vi "Main - bkp 2.vi"() -> ()   [LabVIEW 2013]
uses:
  <vilib>/Utility/error.llb/DialogType.ctl
  <vilib>/Utility/miscctls.llb/LVFontTypeDef.ctl
panel:
  out "TctrlConID":refnum<k5>
  out "Error BuvVIctrl":string[](array[string])
  in  "Num of Buvs":u8
  out "BuvCtrlVI_VIRef":refnum<vi>[](array[refnum])
  out "BuvNameArr":string[](array[string])
  out "Buv IP":string[](array[string])
  out "Buv con ID":refnum<k5>
  out "LoadPhase":bool
  in  "Tab Control":T1(tab)
  in  "List of channels":i32(listbox)
  in  "ReadFromFile":bool
  in  "WriteToFile":bool
  out "Дата":string
  out "Время":string
  in  "Comm. current %":dbl=0.5 caption="А" min=0.0 max=72.0 step=0.25
  in  "Common curr. dec":bool
  in  "Common curr. inc":bool
  in  "ConnectAll":bool
  in  "DisconnectAll":bool
  in  "Set Output ON All":bool caption="ВЫХОДЫ ИСТОЧНИКОВ"
  out "текущий ист.":u8
  in  "SetCurrent":dbl min=0.0 max=72.0 step=0.1 format="%#.1g"
  in  "SetVoltage":dbl min=0.0 max=30.0 step=0.1 format="%#.1g"
  in  "SetCurrentB":bool
  in  "SetVoltageB":bool
  in  "SetOutputOffB":bool
  in  "SetOutputOnB":bool
  in  "ConnectChannel":bool
  in  "DisconnectChannel":bool
  out "Напор \nобщий":dbl
  out "Cлив \nобщий":dbl
  out "K3":dbl
  out "К2":dbl
  out "К1":dbl
  out "T upd fl":bool
  in  "NewBuvName":string caption="Имя"
  in  "NewBuvIP":string="172.16.21.xx" caption="IP"
  in  "DeleteBuv":bool caption="Удалить БУВ"
  out "текущий ист. БУВ":u8
  in  "SelectedBuvOutVolt":dbl min=0.0 max=1000.0 step=0.1 format="%.1f"
  in  "SelectedBuvSetVolB":bool
  in  "Buv Table":i32(listbox)=-1
  in  "Quit":bool=TRUE
  in  "AddNewBuv":bool caption="Добавить БУВ"
  out "message event":string=" INSTRUCTIONS:\r\rNormal Use:  When using subVIs that incorporate the error in/error out (or error I/O) structure, place this handler where you want to inform the user of an error, typically at the end of the I/O data path, as the last action of the program.  If the error in error? is ERROR, the handler creates a message describing the error and its source.  If the type of dialog = 1 (default), the message is displayed to the user, who can only acknowedge it.  If the type = 2, the user can acknowledge the message or abort execution; aborting a program with active I/O is not recommended.  If the type = 0, no message is displayed; this is used to process the error programmatically, and the error out cluster elements are wired to individual terminals for that reason.  \r\rOther Use:\n\r\nlocal testing.  To test the error code of a subVI or function that does not have the error I/O structure, you can wire its error code and a source string to the local error code and error source inputs.  If error in error? indicates no error and error code is not equal to 0, the local code and source are substituted for the error in values, and error? is set TRUE (ERROR)."
  in  "SelectedBuvOutStateB":bool
  out "message upd":string=" INSTRUCTIONS:\r\rNormal Use:  When using subVIs that incorporate the error in/error out (or error I/O) structure, place this handler where you want to inform the user of an error, typically at the end of the I/O data path, as the last action of the program.  If the error in error? is ERROR, the handler creates a message describing the error and its source.  If the type of dialog = 1 (default), the message is displayed to the user, who can only acknowedge it.  If the type = 2, the user can acknowledge the message or abort execution; aborting a program with active I/O is not recommended.  If the type = 0, no message is displayed; this is used to process the error programmatically, and the error out cluster elements are wired to individual terminals for that reason.  \r\rOther Use:\n\r\nlocal testing.  To test the error code of a subVI or function that does not have the error I/O structure, you can wire its error code and a source string to the local error code and error source inputs.  If error in error? indicates no error and error code is not equal to 0, the local code and source are substituted for the error in values, and error? is set TRUE (ERROR)."
  in  "WriteToFile Buv":bool
  in  "ReadFromFile Buv":bool
  in  "SetCurrentAll":bool
  in  "SetVoltageAll":bool
  in  "Comm. voltage %":dbl caption="%" min=0.0 max=100.0 step=0.5
  in  "Common volt. dec":bool
  in  "Common volt. inc":bool
  in  "DeleteChannel":bool
  in  "AddChannel":bool
  out "CURRENTSET":dbl[](array[numeric])
  out "NAME":string[](array[string])
  out "ADRESS":string[](array[string])
  out "Measure_VI":refnum<vi>[](array[refnum])
  # "ВСЕ ИСТОЧНИКИ"
  # "ИСТОЧНИК №_"
  # "Линзы жесткой фокусировки ЛУ-20"
  # "Выбрана линза:"
  # "ЛЖФ"
  # "Система охлаждения\n квадрупольных линз"
  # "ЛУ-20"
  # "°С"
  # "°С"
  # "°С"
  # "°С"
  # "°С"
  # "Бак \nтеплообменника"
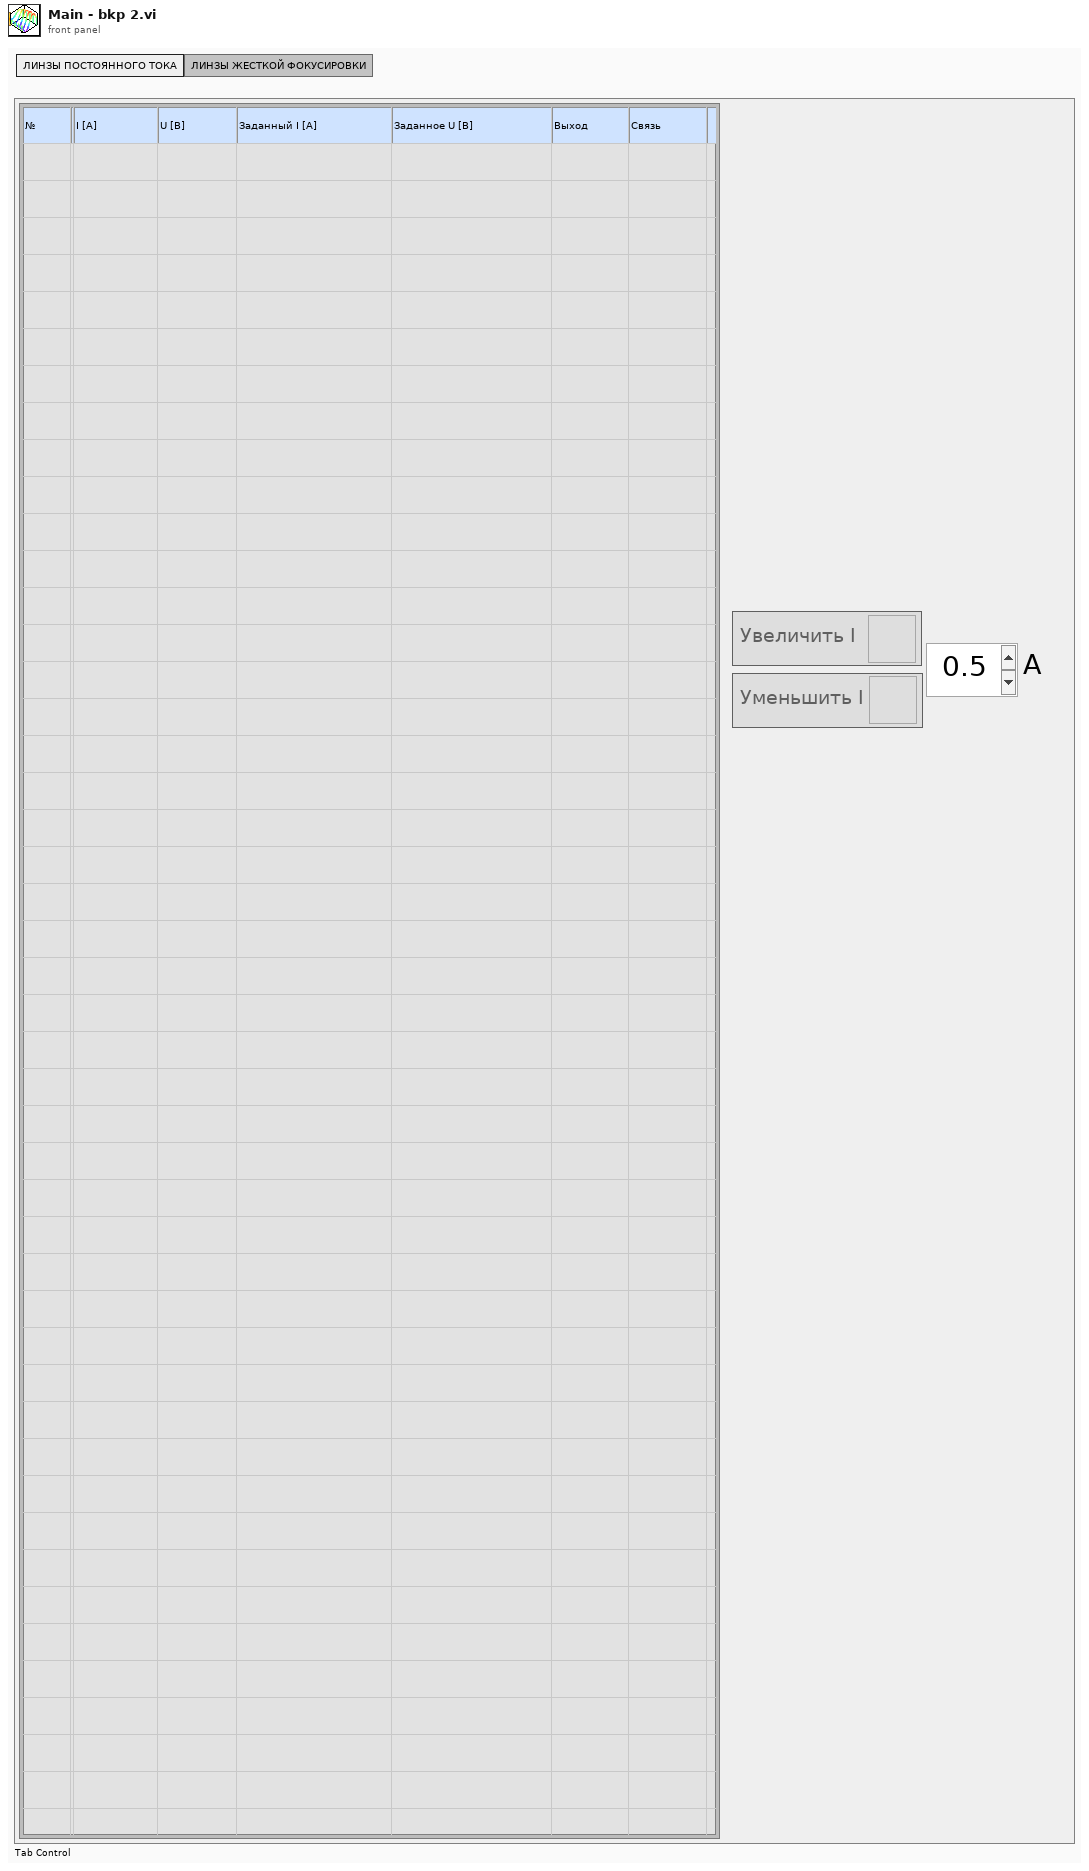
[diagram p1: front panel]
types:
  T1 = enum32{"ЛИНЗЫ ПОСТОЯННОГО ТОКА", "ЛИНЗЫ ЖЕСТКОЙ ФОКУСИРОВКИ"}
  T2 = enum8{"Enabled", "Disabled", "Disabled and Grayed Out"}
  T3 = enum16{"open", "replace", "create", "open or create", "replace or create", "replace or create with confirmation"}
  T4 = typedef "DialogType.ctl" = u16
  T5 = cluster{"T1":dbl, "T2":dbl, "T3":dbl, "T4":dbl, "T5":dbl}
  T6 = cluster{"T 1":bool, "T 2":bool, "T 3":bool, "T 4":bool, "T 5":bool}
  T7 = typedef "LVFontTypeDef.ctl" = cluster{"Font Name":string, "Size":u16, "Bold":bool, "Italic":bool, "Underline":bool, "Strikeout":bool, "Color":u32}
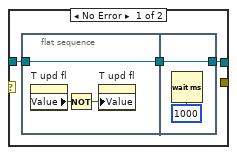
[diagram p2: hidden frame]
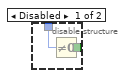
[diagram p4: hidden frame]
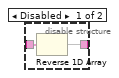
[diagram p6: hidden frame]
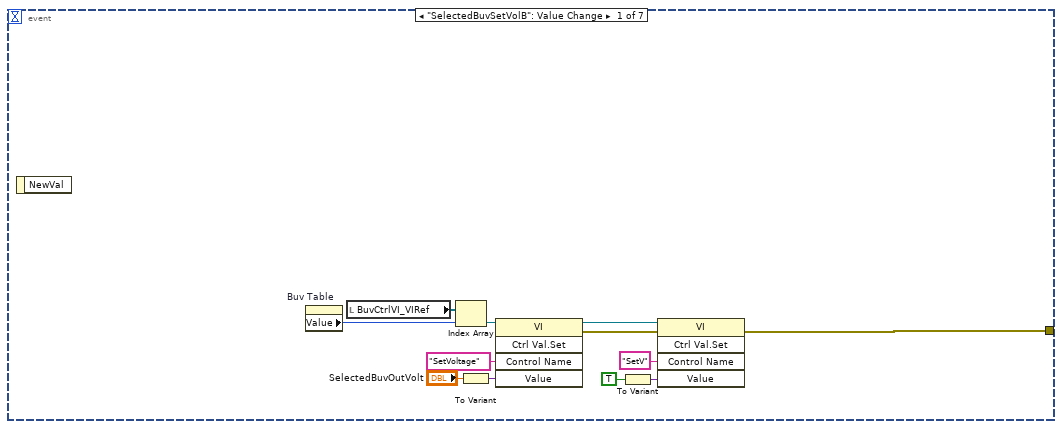
[diagram p7: hidden frame]
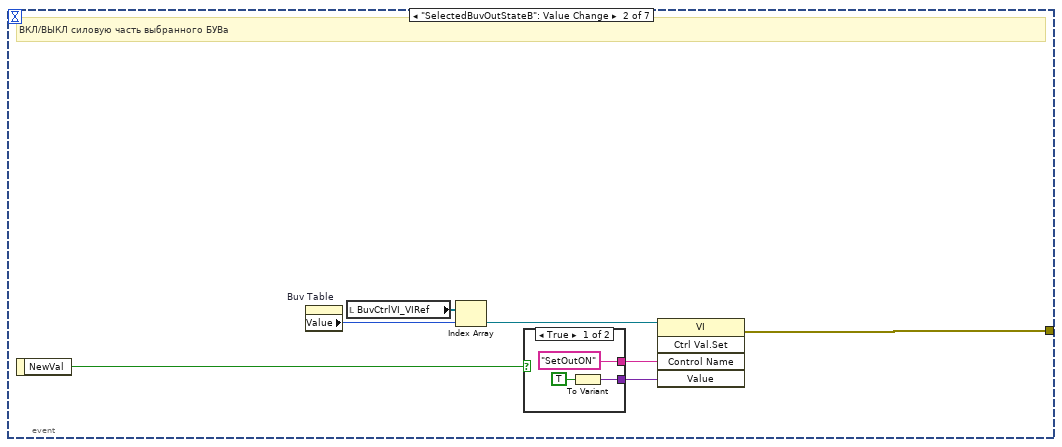
[diagram p8: hidden frame]
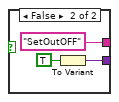
[diagram p9: hidden frame]
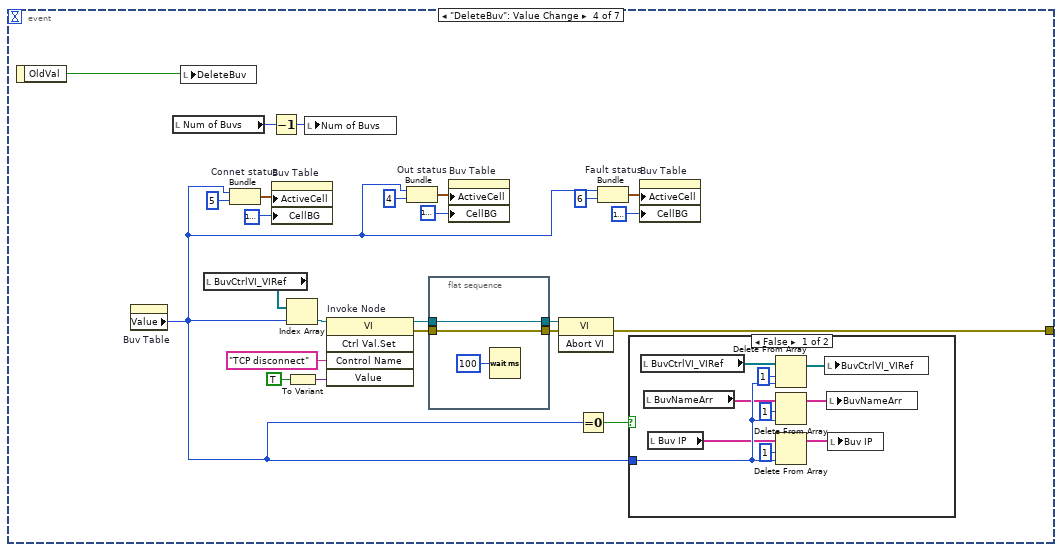
[diagram p10: hidden frame]
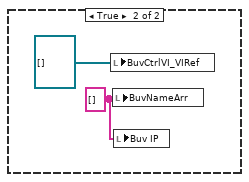
[diagram p11: hidden frame]
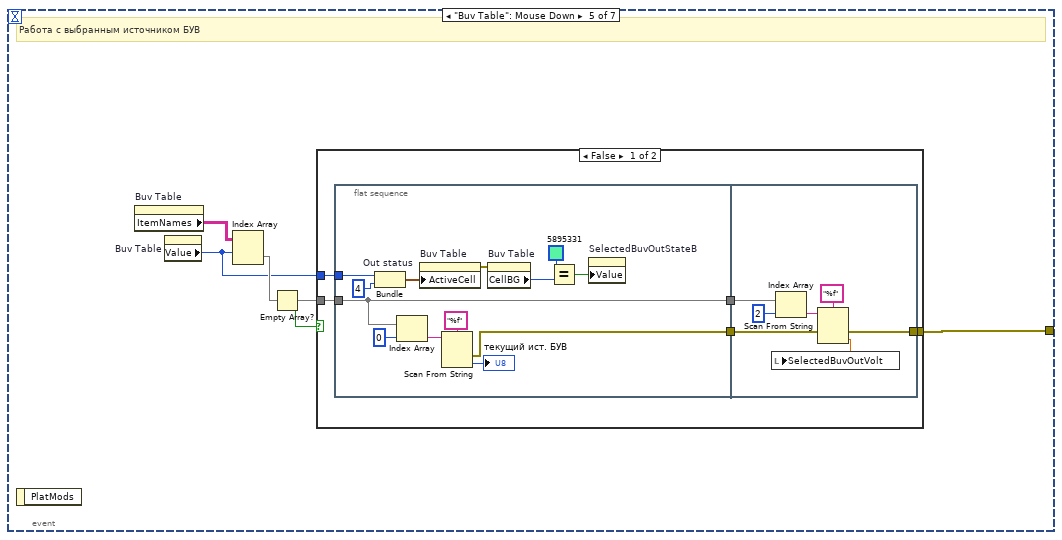
[diagram p12: hidden frame]
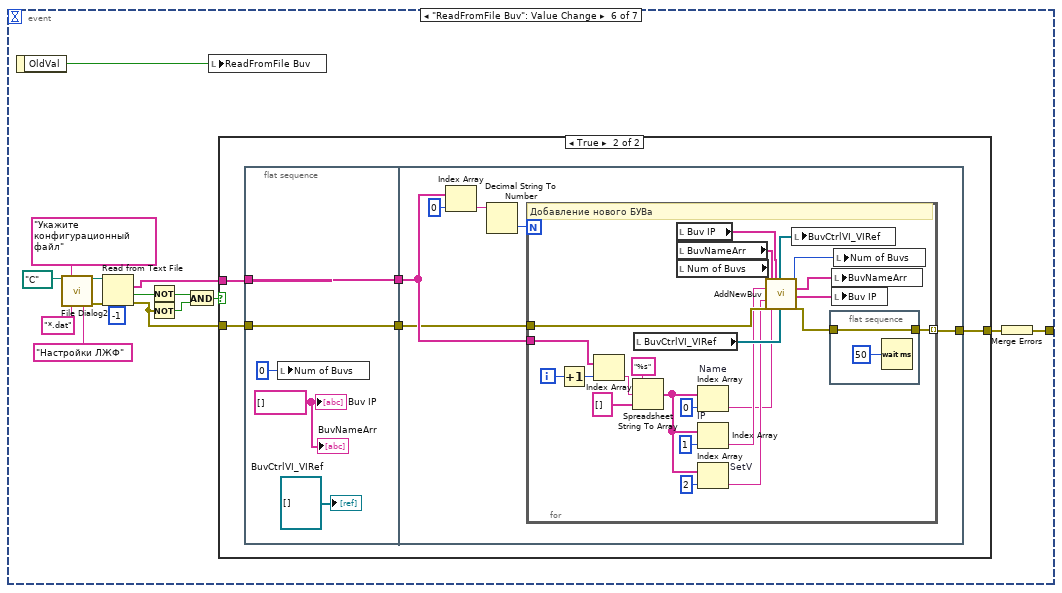
[diagram p14: hidden frame]
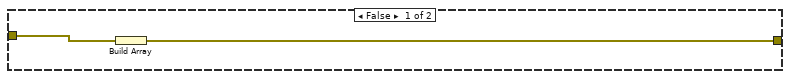
[diagram p15: hidden frame]
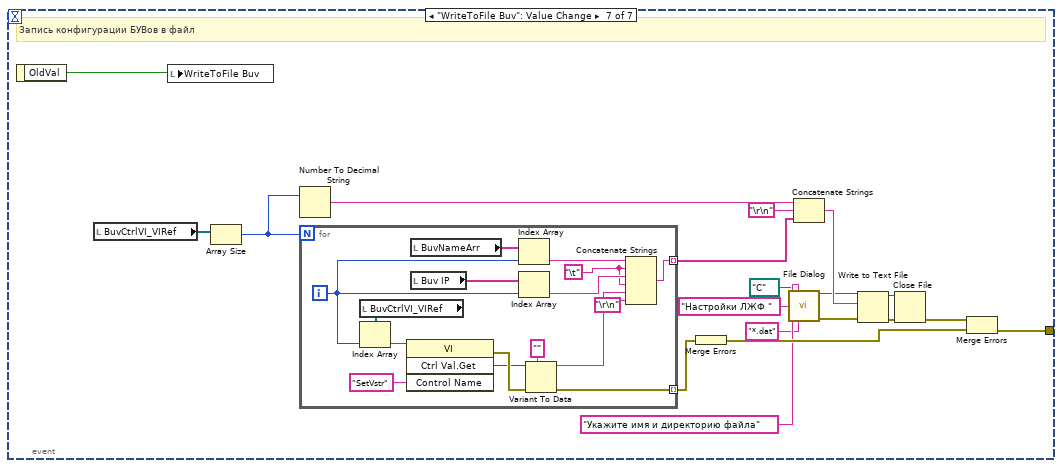
[diagram p16: hidden frame]
diagram:
  w4 = string[] [] ("GlobalInAdress")
  w7 = string[] [] ("GlobalInAdress")
  w24 = u8 0 ("Disabled")
  w8 = FALSE ("SetOutputOnB")
  w26 = FALSE ("OK Button")
  n1 = while {
    stop <- FALSE stop-if-true
    n2 = property on="List of channels" class="MCListbox (strict)"() -> ("ItemNames"=w37:string[][])  [unwired: 2 in, 2 out]
    n3 = Get Date/Time String(want seconds? (F)=TRUE) -> (date string=→"Дата":string, time string=→"Время":string)  [unwired: 2 in]
    n4 = Wait Until Next ms Multiple(millisecond multiple=u16 1000) -> ()  [unwired: 1 out]
    n5 = Empty Array?(array=w37) -> (empty?=w36:bool)
    n6 = case shown="True" w36 {
      tunnel: [T2."Enabled" ("Disabled") T2."Disabled and Grayed Out" ("Disabled")] -> w31
      frame False {
      }
      frame True {
      }
    }
    n7 = property on="Common curr. inc" class="Bool (strict)"("DisabledEnum"=w31) -> ()  [unwired: 2 in, 2 out]
    n8 = property on="Common curr. dec" class="Bool (strict)"("DisabledEnum"=w31) -> ()  [unwired: 2 in, 2 out]
    n9 = property on="Set Output ON All" class="Bool (strict)"("DisabledEnum"=w31) -> ()  [unwired: 2 in, 2 out]
    n10 = property on="Common volt. inc" class="Bool (strict)"("DisabledEnum"=w31) -> ()  [unwired: 2 in, 2 out]
    n11 = property on="DisconnectAll" class="Bool (strict)"("DisabledEnum"=w31) -> ()  [unwired: 2 in, 2 out]
    n12 = property on="SetVoltageB" class="Bool (strict)"("DisabledEnum"=w31) -> ()  [unwired: 2 in, 2 out]
    n13 = property on="ConnectChannel" class="Bool (strict)"("DisabledEnum"=w31) -> ()  [unwired: 2 in, 2 out]
    n14 = property on="SetOutputOnB" class="Bool (strict)"("DisabledEnum"=w31) -> ()  [unwired: 2 in, 2 out]
    n15 = property on="DisconnectChannel" class="Bool (strict)"("DisabledEnum"=w31) -> ()  [unwired: 2 in, 2 out]
    n16 = property on="SetOutputOffB" class="Bool (strict)"("DisabledEnum"=w31) -> ()  [unwired: 2 in, 2 out]
    n17 = property on="ConnectAll" class="Bool (strict)"("DisabledEnum"=w31) -> ()  [unwired: 2 in, 2 out]
    n18 = property on="SetCurrentB" class="Bool (strict)"("DisabledEnum"=w31) -> ()  [unwired: 2 in, 2 out]
  }
  n19 = while {
    stop <- FALSE stop-if-true
    n20 = property on="AddChannel" class="Bool (strict)"() -> ("Disabled"=w48:u8)  [unwired: 2 in, 2 out]
    n21 = Wait Until Next ms Multiple(millisecond multiple=u32 50) -> ()  [unwired: 1 out]
    n22 = local read "Quit"() -> (w46:bool)
    n23 = Not(x=w46) -> (.not. x?=w45:bool)
    n24 = Equal?(x=w48, y=u8 0) -> (x = y?=w44:bool)
    n25 = And(x=w45, y=w44) -> (x .and. y?=w43:bool)
    n26 = case shown="True" w43 {
      frame False {
      }
      frame True {
        w54 = string[] [] ("GlobalInAdress")
        n27 = local read "Measure_VI"() -> (w61:refnum<vi>[])
        n28 = Array Size(array=w61) -> (size(s)=w53:i32)
        n29 = for {
          N: w53 -> [_]
          tunnel: w61 -> [w124]
          shift-right: [w66] -> w52
          shift-left: w54 -> [w63]
          shift-right: [w65] -> w51
          shift-left: w54 -> [w64]
          shift-right: [w115] -> w49
          shift-left: w54 -> [w116]
          shift-right: [w106] -> w50
          shift-left: w54 -> [w111]
          shift-right: [w109] -> w57
          shift-left: w54 -> [w91]
          shift-right: [w104] -> w56
          shift-left: w54 -> [w105]
          i -> [w87]
          w103 = "" ("Control Name")
          n30 = Index Array(array=w124, index=w87) -> (element=w90:refnum<vi>)
          n31 = invoke on="Invoke Node" class="VI" method="Ctrl Val.Get"(reference=w90, "Control Name"="SetVoltageStr") -> (error out=w98:errorcluster, "Get Control Value Variant"=w114:variant)  [unwired: 2 in, 2 out]
          n32 = invoke class="VI" method="Ctrl Val.Get"(reference=w90, "Control Name"="SetCurrentStr") -> (error out=w97:errorcluster, "Get Control Value Variant"=w113:variant)  [unwired: 2 in, 2 out]
          n33 = invoke class="VI" method="Ctrl Val.Get"(reference=w90, "Control Name"="Error") -> (error out=w86:errorcluster, "Get Control Value Variant"=w92:variant)  [unwired: 2 in, 2 out]
          n34 = invoke class="VI" method="Ctrl Val.Get"(reference=w90, "Control Name"="GetCurrent") -> (error out=w100:errorcluster, "Get Control Value Variant"=w121:variant)  [unwired: 2 in, 2 out]
          n35 = invoke class="VI" method="Ctrl Val.Get"(reference=w90, "Control Name"="GetVoltage") -> (error out=w99:errorcluster, "Get Control Value Variant"=w122:variant)  [unwired: 2 in, 2 out]
          n36 = invoke class="VI" method="Ctrl Val.Get"(reference=w90, "Control Name"="Output") -> (error out=w96:errorcluster, "Get Control Value Variant"=w107:variant)  [unwired: 2 in, 2 out]
          n37 = Variant To Data(type=w103, Variant=w114) -> (data=w68:string)  [unwired: 1 in, 1 out]
          n38 = Variant To Data(type=w103, Variant=w113) -> (data=w73:string)  [unwired: 1 in, 1 out]
          n39 = Merge Errors(w86, w100, w99, w98) -> (w95:errorcluster)
          n40 = Variant To Data(type=w103, Variant=w121) -> (data=w118:string)  [unwired: 1 in, 1 out]
          n41 = Variant To Data(type=w103, Variant=w122) -> (data=w119:string)  [unwired: 1 in, 1 out]
          n42 = Variant To Data "Out"(type=w103, Variant=w107) -> (data=w93:string)  [unwired: 1 in, 1 out]
          n43 = Merge Errors(w97, w96) -> (w94:errorcluster)
          n44 = String Length(string=w68) -> (length=w69:i32)
          n45 = String Length(string=w73) -> (length=w76:i32)
          n46 = Variant To Data(type=FALSE, Variant=w92) -> (data=w62:bool)  [unwired: 1 in, 1 out]
          n47 = case shown="False" w62 {
            tunnel: w90 -> [_ w178]
            tunnel: w87 -> [w165 w171]
            tunnel: [w164 w169] -> w83
            frame False {
              n48 = Bundle(w165, "milliseconds to wait"=8) -> (w166:cluster{i32, "milliseconds to wait":i32})  [unwired: 1 in]
              n49 = property on="error" class="MCListbox (strict)"("ActiveCell"=w166, "CellBG"=u32 16777225) -> (error out=w164:errorcluster)  [unwired: 2 in, 1 out]
            }
            frame True {
              n50 = disable-structure shown="Enabled" {
                disable-tunnel: w178 -> [w194 w200]
                disable-tunnel: [w191 _] -> w174
                disable-tunnel: [w189 w200] -> w173
                disable-tunnel: [w187 _] -> w172
                disable-tunnel: w171 -> [w186 w201]
                disable-tunnel: [w185 w201] -> w170
                frame Disabled {
                  w188 = "Connect" ("Control Name")
                  n51 = invoke class="VI" method="Ctrl Val.Set"(reference=w194, "Control Name"=w188, "Value"=FALSE ("OK Button")) -> (reference out=w190:refnum<vi>, error out=w192:errorcluster)  [unwired: 2 in, 3 out]
                  n52 = flat-sequence {
                    tunnel: w192 -> [w199]
                    tunnel: [w199] -> w191
                    tunnel: w190 -> [w197]
                    tunnel: [w197] -> w189
                    tunnel: w188 -> [w196]
                    tunnel: [w196] -> w187
                    tunnel: w186 -> [w195]
                    tunnel: [w195] -> w185
                    frame #0 {
                      n53 = Wait (ms)(milliseconds to wait=u32 2000) -> ()  [unwired: 1 out]
                    }
                  }
                }
                frame Enabled {
                }
              }
              n54 = disable-structure shown="Enabled" {
                disable-tunnel: w174 -> [w182 w184]
                disable-tunnel: w173 -> [w181 _]
                disable-tunnel: w172 -> [w180 _]
                disable-tunnel: [w179 w184] -> w169
                frame Disabled {
                  n55 = invoke class="VI" method="Ctrl Val.Set"(reference=w181, error in=w182, "Control Name"=w180, "Value"=TRUE ("OK Button")) -> (error out=w179:errorcluster)  [unwired: 1 in, 4 out]
                }
                frame Enabled {
                }
              }
              n56 = Bundle(w170, "milliseconds to wait"=8) -> (w175:cluster{i32, "milliseconds to wait":i32})  [unwired: 1 in]
              n57 = property on="error" class="MCListbox (strict)"("ActiveCell"=w175, "CellBG"=u32 16711680) -> ()  [unwired: 2 in, 2 out]
            }
          }
          n58 = case shown="6, Default" w69 {
            tunnel: [4 ("milliseconds to wait") 5 ("milliseconds to wait")] -> w70
            tunnel: [0 ("milliseconds to wait") 0 ("milliseconds to wait")] -> w71
            frame 6, Default {
            }
            frame 7 {
            }
          }
          n59 = case shown="7" w76 {
            tunnel: [4 ("milliseconds to wait") 5 ("milliseconds to wait")] -> w75
            tunnel: [0 ("milliseconds to wait") 0 ("milliseconds to wait")] -> w74
            frame 6, Default {
            }
            frame 7 {
            }
          }
          n60 = Build Array (concatenate)(w63, w118) -> (w66:string[])
          n61 = Build Array (concatenate)(w64, w119) -> (w65:string[])
          n62 = Merge Errors(w95, w94, w83) -> (w89:errorcluster)
          n63 = call <vilib>:"General Error Handler.vi"("type of dialog (OK msg:1)"=u32 0 ("milliseconds to wait"), "error in (no error)"=w89) -> ()  [unwired: 9 in, 5 out]
          n64 = case shown="\"0\"" w93 {
            tunnel: ["+" ("Control Name") "" ("Control Name") "-" ("Control Name")] -> w85
            tunnel: w87 -> [w133 w138 w143]
            frame "1" {
              n65 = Bundle(w133, "milliseconds to wait"=6) -> (w135:cluster{i32, "milliseconds to wait":i32})  [unwired: 1 in]
              n66 = property on="out" class="MCListbox (strict)"("ActiveCell"=w135, "CellBG"=u32 5895331) -> ()  [unwired: 2 in, 2 out]
            }
            frame Default {
              n67 = Bundle(w138, "milliseconds to wait"=6) -> (w140:cluster{i32, "milliseconds to wait":i32})  [unwired: 1 in]
              n68 = property on="out" class="MCListbox (strict)"("ActiveCell"=w140, "CellBG"=u32 16777225) -> ()  [unwired: 2 in, 2 out]
            }
            frame "0" {
              n69 = Bundle(w143, "milliseconds to wait"=6) -> (w145:cluster{i32, "milliseconds to wait":i32})  [unwired: 1 in]
              n70 = property on="out" class="MCListbox (strict)"("ActiveCell"=w145, "CellBG"=u32 13816530) -> ()  [unwired: 2 in, 2 out]
            }
          }
          n71 = String Subset(string=w68, offset (0)=w71, length (rest)=w70) -> (substring=w67:string)
          n72 = String Subset(string=w73, offset (0)=w74, length (rest)=w75) -> (substring=w72:string)
          n73 = case shown="False" w62 {
            tunnel: ["+" ("Control Name") "-" ("Control Name")] -> w110
            tunnel: w87 -> [w149 w156]
            tunnel: w85 -> [w148 _]
            tunnel: [w148 "?" ("Control Name")] -> w84
            frame False {
              n74 = Bundle(w149, "milliseconds to wait"=7) -> (w151:cluster{i32, "milliseconds to wait":i32})  [unwired: 1 in]
              n75 = property on="active" class="MCListbox (strict)"("ActiveCell"=w151, "CellBG"=u32 5895331) -> ()  [unwired: 2 in, 2 out]
            }
            frame True {
              n76 = Bundle(w156, "milliseconds to wait"=7) -> (w162:cluster{i32, "milliseconds to wait":i32})  [unwired: 1 in]
              n77 = property on="active" class="MCListbox (strict)"("ActiveCell"=w162, "CellBG"=u32 14869218) -> (error out=w157:errorcluster)  [unwired: 2 in, 1 out]
              n78 = Bundle(w156, "milliseconds to wait"=6) -> (w155:cluster{i32, "milliseconds to wait":i32})  [unwired: 1 in]
              n79 = property on="out" class="MCListbox (strict)"(error in=w157, "ActiveCell"=w155, "CellBG"=u32 14869218) -> ()  [unwired: 1 in, 2 out]
            }
          }
          n80 = Search and Replace String(input string=w67, search string=",", replace string="." ("replace string (\"\")")) -> (result string=w80:string)  [unwired: 5 in, 3 out]
          n81 = Search and Replace String(input string=w72, search string=",", replace string="." ("replace string (\"\")")) -> (result string=w78:string)  [unwired: 5 in, 3 out]
          n82 = Build Array (concatenate)(w111, w78) -> (w106:string[])
          n83 = Build Array (concatenate)(w116, w80) -> (w115:string[])
          n84 = Build Array (concatenate)(w105, w84) -> (w104:string[])
          n85 = Build Array (concatenate)(w91, w110) -> (w109:string[])
        }
        n86 = local read "ADRESS"() -> (w59:string[])
        n87 = local read "NAME"() -> (w58:string[])
        n88 = Build Array(w58, w59, w52, w51, w50, w49, w56, w57) -> (w60:string[][])
        n89 = Transpose 2D Array(2D array=w60) -> (transposed array=w55:string[][])
        n90 = property on="List of channels" class="MCListbox (strict)"("ItemNames"=w55) -> ()  [unwired: 2 in, 2 out]
      }
    }
  }
  n91 = while {
    stop <- FALSE stop-if-true
    n92 = event shown="[14] \"WriteToFile\": Value Change" {
      selector: _ -> [_ _ _ _ _ _ _ _ _ _ _ _ _ _ _ _ _ _]
      dyn-events: _ -> [_ _ _ _ _ _ _ _ _ _ _ _ _ _ _ _ _ _]
      timeout: _ -> [_ _ _ _ _ _ _ _ _ _ _ _ _ _ _ _ _ _]
      tunnel: [_ _ w272 w288 w304 w345 w386 w401 w427 w443 w459 w476 w497 w520 w538 w589 w667 w690] -> w203
      event "List of channels": Mouse Down {
        # "Работа с выбранным источником"
        n93 = event-data() -> ()  [unwired: 2 out]
        n94 = property on="List of channels" class="MCListbox (strict)"() -> ("ItemNames"=w209:string[][])  [unwired: 2 in, 2 out]
        n95 = property on="List of channels" class="MCListbox (strict)"() -> ("Value"=w208:i32)  [unwired: 2 in, 2 out]
        n96 = Index Array(array=w209, index (row)=w208) -> (element=w207:string[])  [unwired: 1 in]
        n97 = Empty Array?(array=w207) -> (empty?=w206:bool)
        n98 = case shown="False" w206 {
          tunnel: w207 -> [w210 _]
          frame False {
            n99 = flat-sequence {
              tunnel: w210 -> [w216]
              tunnel: [w216] -> w211
              tunnel: w211 -> [w229]
              frame #0 {
                n100 = Index Array(array=w216, index=0) -> (element=w219:string)
                n101 = Index Array(array=w216, index=7) -> (element=w217:string)
                n102 = case shown="\"-\", Default" w217 {
                  tunnel: [T2."Enabled" ("Disabled") T2."Disabled and Grayed Out" ("Disabled")] -> w212
                  tunnel: [w223 w225] -> w213
                  tunnel: [w223 w225] -> w215
                  tunnel: [w223 w225] -> w214
                  frame "-", Default {
                    w223 = T2."Disabled and Grayed Out" ("Disabled")
                  }
                  frame "+" {
                    w225 = T2."Enabled" ("Disabled")
                    # "соединение с ист."
                  }
                }
                n103 = Scan From String(format string="%f", input string=w219) -> (output 1=→"текущий ист.":u8)  [unwired: 3 in, 3 out]
                n104 = property on="DisconnectAll" class="Bool (strict)"("DisabledEnum"=w213) -> ()  [unwired: 2 in, 2 out]
                n105 = property on="DisconnectChannel" class="Bool (strict)"("DisabledEnum"=w213) -> ()  [unwired: 2 in, 2 out]
                n106 = property on="SetOutputOffB" class="Bool (strict)"("DisabledEnum"=w215) -> ()  [unwired: 2 in, 2 out]
                n107 = property on="SetOutputOnB" class="Bool (strict)"("DisabledEnum"=w214) -> ()  [unwired: 2 in, 2 out]
                n108 = property on="ConnectChannel" class="Bool (strict)"("DisabledEnum"=w212) -> ()  [unwired: 2 in, 2 out]
                n109 = property on="ConnectAll" class="Bool (strict)"("DisabledEnum"=w212) -> ()  [unwired: 2 in, 2 out]
              }
              frame #1 {
                n110 = Index Array(array=w229, index=5) -> (element=w234:string)
                n111 = Index Array(array=w229, index=6) -> (element=w237:string)
                n112 = Index Array(array=w229, index=4) -> (element=w231:string)
                n113 = case shown="\"-\", Default" w237 {
                  tunnel: [T2."Enabled" ("Disabled") T2."Disabled and Grayed Out" ("Disabled") w244] -> w238
                  tunnel: [T2."Disabled and Grayed Out" ("Disabled") T2."Enabled" ("Disabled") w244] -> w239
                  frame "-", Default {
                  }
                  frame "+" {
                  }
                  frame "?" {
                    w244 = T2."Disabled and Grayed Out" ("Disabled")
                  }
                }
                n114 = Scan From String(format string="%f", input string=w234) -> (output 1=w227:dbl)  [unwired: 3 in, 3 out]
                n115 = Scan From String(format string="%f", input string=w231) -> (output 1=w228:dbl)  [unwired: 3 in, 3 out]
                n116 = local write "SetVoltage"(w227) -> ()
                n117 = local write "SetCurrent"(w228) -> ()
                n118 = property on="SetOutputOffB" class="Bool (strict)"("DisabledEnum"=w239) -> ()  [unwired: 2 in, 2 out]
                n119 = property on="SetOutputOnB" class="Bool (strict)"("DisabledEnum"=w238) -> ()  [unwired: 2 in, 2 out]
              }
            }
          }
          frame True {
          }
        }
      }
      event Panel Close? {
        n120 = event-data() -> ()  [unwired: 5 out]
        n121 = Two Button Dialog(message="Вы уверены, что хотите закрыть программу?", 1:"Нет" ("F button name (\"Cancel\")"), 2:"Да" ("T button name (\"OK\")")) -> (T button?=w248:bool)
        n122 = case shown="True" w248 {
          frame False {
          }
          frame True {
            n123 = disable-structure shown="Disabled" {
              frame Disabled {
                n124 = local read item#-1() -> (w258)
                n125 = TCP Close Connection(connection ID=w258) -> ()  [unwired: 2 in, 2 out]
              }
              frame Enabled {
              }
            }
            n126 = local read "Measure_VI"() -> (w250:refnum<vi>[])
            n127 = Array Size(array=w250) -> (size(s)=w249:i32)
            n128 = for {
              N: w249 -> [_]
              tunnel: w250 -> [w268]
              tunnel: [w266] -> w257 mode=indexing
              i -> [w269]
              n129 = Index Array(array=w268, index=w269) -> (element=w267:refnum<vi>)
              n130 = invoke class="VI" method="Ctrl Val.Set"(reference=w267, "Control Name"="Connect", "Value"=FALSE) -> (error out=w266:errorcluster)  [unwired: 2 in, 4 out]
            }
            n131 = flat-sequence {
              tunnel: [w260] -> w256
              tunnel: w257 -> [w260]
              frame #0 {
                n132 = Wait (ms)(milliseconds to wait=u32 1000) -> ()  [unwired: 1 out]
              }
            }
            n133 = local read "Measure_VI"() -> (w251:refnum<vi>[])
            n134 = Array Size(array=w251) -> (size(s)=w252:i32)
            n135 = for {
              N: w252 -> [_]
              tunnel: w251 -> [w264]
              tunnel: [w262] -> w253 mode=indexing
              tunnel: w256 -> [w261] mode=indexing
              i -> [w265]
              n136 = Index Array(array=w264, index=w265) -> (element=w263:refnum<vi>)
              n137 = invoke class="VI" method="Abort VI"(reference=w263, error in=w261) -> (error out=w262:errorcluster)  [unwired: 1 in, 2 out]
            }
            n138 = Merge Errors(w253) -> (w254:errorcluster)
            n139 = call <vilib>:"General Error Handler.vi"("type of dialog (OK msg:1)"=u32 0 ("milliseconds to wait"), "error in (no error)"=w254) -> ()  [unwired: 9 in, 5 out]
          }
        }
        n140 = event-data() -> ()  [unwired: 2 in, 1 out]
      }
      event "SetVoltageAll": Value Change {
        n141 = event-data() -> ()  [unwired: 7 out]
        n142 = flat-sequence {
          tunnel: [w276] -> w274
          tunnel: [w285] -> w273
          tunnel: w274 -> [w285]
          frame #0 {
            w275 = u8 2 ("Disabled")
            n143 = property on="Quit" class="Bool (strict)"("Disabled"=w275) -> ()  [unwired: 2 in, 2 out]
            n144 = property on="AddChannel" class="Bool (strict)"("Disabled"=w275) -> ()  [unwired: 2 in, 2 out]
            n145 = property on="DisconnectChannel" class="Bool (strict)"("Disabled"=w275) -> ()  [unwired: 2 in, 2 out]
            n146 = property on="ConnectAll" class="Bool (strict)"("Disabled"=w275) -> ()  [unwired: 2 in, 2 out]
            n147 = property on="ReadFromFile" class="Bool (strict)"("Disabled"=w275) -> ()  [unwired: 2 in, 2 out]
            n148 = property on="ConnectChannel" class="Bool (strict)"("Disabled"=w275) -> ()  [unwired: 2 in, 2 out]
            n149 = property on="DeleteChannel" class="Bool (strict)"("Disabled"=w275) -> ()  [unwired: 2 in, 2 out]
            n150 = property on="SetVoltageB" class="Bool (strict)"("Disabled"=w275) -> ()  [unwired: 2 in, 2 out]
            n151 = property on="Set Output ON All" class="Bool (strict)"("Disabled"=w275) -> ()  [unwired: 2 in, 2 out]
            n152 = property on="SetOutputOffB" class="Bool (strict)"("Disabled"=w275) -> ()  [unwired: 2 in, 2 out]
            n153 = property on="SetVoltageAll" class="Bool (strict)"("Disabled"=w275) -> ()  [unwired: 2 in, 2 out]
            n154 = property on="SetCurrentAll" class="Bool (strict)"("Disabled"=w275) -> ()  [unwired: 2 in, 2 out]
            n155 = property on="DisconnectAll" class="Bool (strict)"("Disabled"=w275) -> ()  [unwired: 2 in, 2 out]
            n156 = property on="WriteToFile" class="Bool (strict)"("Disabled"=w275) -> ()  [unwired: 2 in, 2 out]
            n157 = property on="SetCurrentB" class="Bool (strict)"("Disabled"=w275) -> ()  [unwired: 2 in, 2 out]
            n158 = property on="SetOutputOnB" class="Bool (strict)"("Disabled"=w275) -> ()  [unwired: 2 in, 2 out]
          }
          frame #1 {
            n159 = local read "Measure_VI"() -> (w278:refnum<vi>[])
            n160 = Array Size(array=w278) -> (size(s)=w277:i32)
            n161 = for {
              N: w277 -> [_]
              tunnel: [w279] -> w276 mode=indexing
              i -> [w281]
              n162 = local read "Measure_VI"() -> (w284:refnum<vi>[])
              n163 = Index Array(array=w284, index=w281) -> (element=w280:refnum<vi>)
              n164 = invoke class="VI" method="Ctrl Val.Set"(reference=w280, "Control Name"="NeedToSetVoltage", "Value"=TRUE ("ConnectChannel")) -> (error out=w279:errorcluster)  [unwired: 2 in, 4 out]
            }
          }
          frame #2 {
            w286 = u8 0 ("Disabled")
            n165 = local write "SetVoltageAll"(FALSE ("SetVoltageAll")) -> ()
            n166 = property on="Quit" class="Bool (strict)"("Disabled"=w286) -> ()  [unwired: 2 in, 2 out]
            n167 = property on="AddChannel" class="Bool (strict)"("Disabled"=w286) -> ()  [unwired: 2 in, 2 out]
            n168 = property on="DisconnectChannel" class="Bool (strict)"("Disabled"=w286) -> ()  [unwired: 2 in, 2 out]
            n169 = property on="ReadFromFile" class="Bool (strict)"("Disabled"=w286) -> ()  [unwired: 2 in, 2 out]
            n170 = property on="ConnectChannel" class="Bool (strict)"("Disabled"=w286) -> ()  [unwired: 2 in, 2 out]
            n171 = property on="DeleteChannel" class="Bool (strict)"("Disabled"=w286) -> ()  [unwired: 2 in, 2 out]
            n172 = property on="WriteToFile" class="Bool (strict)"("Disabled"=w286) -> ()  [unwired: 2 in, 2 out]
            n173 = property on="Set Output ON All" class="Bool (strict)"("Disabled"=w286) -> ()  [unwired: 2 in, 2 out]
            n174 = property on="SetCurrentB" class="Bool (strict)"("Disabled"=w286) -> ()  [unwired: 2 in, 2 out]
            n175 = property on="ConnectAll" class="Bool (strict)"("Disabled"=w286) -> ()  [unwired: 2 in, 2 out]
            n176 = property on="SetOutputOnB" class="Bool (strict)"("Disabled"=w286) -> ()  [unwired: 2 in, 2 out]
            n177 = property on="SetVoltageB" class="Bool (strict)"("Disabled"=w286) -> ()  [unwired: 2 in, 2 out]
            n178 = property on="SetOutputOffB" class="Bool (strict)"("Disabled"=w286) -> ()  [unwired: 2 in, 2 out]
            n179 = property on="SetVoltageAll" class="Bool (strict)"("Disabled"=w286) -> ()  [unwired: 2 in, 2 out]
            n180 = property on="SetCurrentAll" class="Bool (strict)"("Disabled"=w286) -> ()  [unwired: 2 in, 2 out]
            n181 = property on="DisconnectAll" class="Bool (strict)"("Disabled"=w286) -> ()  [unwired: 2 in, 2 out]
          }
        }
        n182 = Merge Errors(w273) -> (w272:errorcluster)
      }
      event "SetCurrentAll": Value Change {
        n183 = event-data() -> ()  [unwired: 7 out]
        n184 = flat-sequence {
          tunnel: [w292] -> w290
          tunnel: [w301] -> w289
          tunnel: w290 -> [w301]
          frame #0 {
            w291 = u8 2 ("Disabled")
            n185 = property on="Quit" class="Bool (strict)"("Disabled"=w291) -> ()  [unwired: 2 in, 2 out]
            n186 = property on="AddChannel" class="Bool (strict)"("Disabled"=w291) -> ()  [unwired: 2 in, 2 out]
            n187 = property on="DisconnectChannel" class="Bool (strict)"("Disabled"=w291) -> ()  [unwired: 2 in, 2 out]
            n188 = property on="ConnectAll" class="Bool (strict)"("Disabled"=w291) -> ()  [unwired: 2 in, 2 out]
            n189 = property on="ReadFromFile" class="Bool (strict)"("Disabled"=w291) -> ()  [unwired: 2 in, 2 out]
            n190 = property on="ConnectChannel" class="Bool (strict)"("Disabled"=w291) -> ()  [unwired: 2 in, 2 out]
            n191 = property on="DeleteChannel" class="Bool (strict)"("Disabled"=w291) -> ()  [unwired: 2 in, 2 out]
            n192 = property on="SetOutputOffB" class="Bool (strict)"("Disabled"=w291) -> ()  [unwired: 2 in, 2 out]
            n193 = property on="Set Output ON All" class="Bool (strict)"("Disabled"=w291) -> ()  [unwired: 2 in, 2 out]
            n194 = property on="SetVoltageAll" class="Bool (strict)"("Disabled"=w291) -> ()  [unwired: 2 in, 2 out]
            n195 = property on="SetCurrentAll" class="Bool (strict)"("Disabled"=w291) -> ()  [unwired: 2 in, 2 out]
            n196 = property on="DisconnectAll" class="Bool (strict)"("Disabled"=w291) -> ()  [unwired: 2 in, 2 out]
            n197 = property on="WriteToFile" class="Bool (strict)"("Disabled"=w291) -> ()  [unwired: 2 in, 2 out]
            n198 = property on="SetCurrentB" class="Bool (strict)"("Disabled"=w291) -> ()  [unwired: 2 in, 2 out]
            n199 = property on="SetOutputOnB" class="Bool (strict)"("Disabled"=w291) -> ()  [unwired: 2 in, 2 out]
            n200 = property on="SetVoltageB" class="Bool (strict)"("Disabled"=w291) -> ()  [unwired: 2 in, 2 out]
          }
          frame #1 {
            n201 = local read "Measure_VI"() -> (w294:refnum<vi>[])
            n202 = Array Size(array=w294) -> (size(s)=w293:i32)
            n203 = for {
              N: w293 -> [_]
              tunnel: [w295] -> w292 mode=indexing
              i -> [w297]
              n204 = local read "Measure_VI"() -> (w300:refnum<vi>[])
              n205 = Index Array(array=w300, index=w297) -> (element=w296:refnum<vi>)
              n206 = invoke class="VI" method="Ctrl Val.Set"(reference=w296, "Control Name"="NeedToSetCurrent", "Value"=TRUE ("ConnectChannel")) -> (error out=w295:errorcluster)  [unwired: 2 in, 4 out]
            }
          }
          frame #2 {
            w302 = u8 0 ("Disabled")
            n207 = local write "SetCurrentAll"(FALSE ("SetVoltageAll")) -> ()
            n208 = property on="Quit" class="Bool (strict)"("Disabled"=w302) -> ()  [unwired: 2 in, 2 out]
            n209 = property on="AddChannel" class="Bool (strict)"("Disabled"=w302) -> ()  [unwired: 2 in, 2 out]
            n210 = property on="DisconnectChannel" class="Bool (strict)"("Disabled"=w302) -> ()  [unwired: 2 in, 2 out]
            n211 = property on="ReadFromFile" class="Bool (strict)"("Disabled"=w302) -> ()  [unwired: 2 in, 2 out]
            n212 = property on="ConnectChannel" class="Bool (strict)"("Disabled"=w302) -> ()  [unwired: 2 in, 2 out]
            n213 = property on="DeleteChannel" class="Bool (strict)"("Disabled"=w302) -> ()  [unwired: 2 in, 2 out]
            n214 = property on="WriteToFile" class="Bool (strict)"("Disabled"=w302) -> ()  [unwired: 2 in, 2 out]
            n215 = property on="Set Output ON All" class="Bool (strict)"("Disabled"=w302) -> ()  [unwired: 2 in, 2 out]
            n216 = property on="SetCurrentB" class="Bool (strict)"("Disabled"=w302) -> ()  [unwired: 2 in, 2 out]
            n217 = property on="ConnectAll" class="Bool (strict)"("Disabled"=w302) -> ()  [unwired: 2 in, 2 out]
            n218 = property on="SetOutputOnB" class="Bool (strict)"("Disabled"=w302) -> ()  [unwired: 2 in, 2 out]
            n219 = property on="SetVoltageB" class="Bool (strict)"("Disabled"=w302) -> ()  [unwired: 2 in, 2 out]
            n220 = property on="SetOutputOffB" class="Bool (strict)"("Disabled"=w302) -> ()  [unwired: 2 in, 2 out]
            n221 = property on="SetVoltageAll" class="Bool (strict)"("Disabled"=w302) -> ()  [unwired: 2 in, 2 out]
            n222 = property on="SetCurrentAll" class="Bool (strict)"("Disabled"=w302) -> ()  [unwired: 2 in, 2 out]
            n223 = property on="DisconnectAll" class="Bool (strict)"("Disabled"=w302) -> ()  [unwired: 2 in, 2 out]
          }
        }
        n224 = Merge Errors(w289) -> (w288:errorcluster)
      }
      event "Common curr. inc", "Common curr. dec": Value Change {
        # "Увелич/уменьшение тока на всех ист"
        n225 = event-data() -> ()  [unwired: 2 out]
        n226 = local read "ADRESS"() -> (w307:string[])
        n227 = Array Size(array=w307) -> (size(s)=w308:i32)
        n228 = for {
          N: w308 -> [_]
          tunnel: [w318] -> w306 mode=indexing
          i -> [w332]
          n229 = local read "Measure_VI"() -> (w335:refnum<vi>[])
          n230 = Index Array(array=w335, index=w332) -> (element=w326:refnum<vi>)
          n231 = invoke class="VI" method="Ctrl Val.Get"(reference=w326, "Control Name"="SetCurrentStr") -> (reference out=w320:refnum<vi>, error out=w330:errorcluster, "Get Control Value Variant"=w334:variant)  [unwired: 2 in, 1 out]
          n232 = Variant To Data(error in=w330, type="" ("Control Name"), Variant=w334) -> (data=w329:string, error out=w328:errorcluster)
          n233 = Scan From String(format string="%f", input string=w329, error in=w328) -> (error out=w319:errorcluster, output 1=w317:dbl)  [unwired: 2 in, 2 out]
          n234 = local read "Common curr. inc"() -> (w316:bool)
          n235 = local read "Common curr. dec"() -> (w314:bool)
          n236 = case shown="True" w316 {
            tunnel: "Comm. current %" -> [w340 w344]
            tunnel: w317 -> [w341 w343]
            tunnel: [w341 w342] -> w315
            tunnel: [w340 _] -> w313
            frame False {
            }
            frame True {
              n237 = Add(x=w343, y=w344) -> (x+y=w342:dbl)
            }
          }
          n238 = case shown="True" w314 {
            tunnel: w315 -> [w336 w339]
            tunnel: [w336 w338] -> w312
            tunnel: w313 -> [_ w337]
            frame False {
            }
            frame True {
              n239 = Subtract(x=w339, y=w337) -> (x-y=w338:dbl)
            }
          }
          n240 = invoke class="VI" method="Ctrl Val.Set"(reference=w320, error in=w319, "Control Name"="SetCurrent", "Value"=w312) -> (reference out=w322:refnum<vi>, error out=w321:errorcluster)  [unwired: 1 in, 3 out]
          n241 = invoke class="VI" method="Ctrl Val.Set"(reference=w322, error in=w321, "Control Name"="NeedToSetCurrent", "Value"=TRUE ("ConnectChannel")) -> (error out=w318:errorcluster)  [unwired: 1 in, 4 out]
        }
        n242 = Merge Errors(w306) -> (w305:errorcluster)
        n243 = flat-sequence {
          tunnel: w305 -> [w310]
          tunnel: [w310] -> w304
          frame #0 {
            w309 = FALSE ("ConnectChannel")
            n244 = local write "Common curr. inc"(w309) -> ()
            n245 = local write "Common curr. dec"(w309) -> ()
          }
        }
      }
      event "Common volt. inc", "Common volt. dec": Value Change {
        # "Увелич/уменьшение тока на всех ист"
        n246 = event-data() -> ()  [unwired: 2 out]
        n247 = local read "ADRESS"() -> (w348:string[])
        n248 = Array Size(array=w348) -> (size(s)=w349:i32)
        n249 = for {
          N: w349 -> [_]
          tunnel: [w359] -> w347 mode=indexing
          i -> [w373]
          n250 = local read "Measure_VI"() -> (w376:refnum<vi>[])
          n251 = Index Array(array=w376, index=w373) -> (element=w367:refnum<vi>)
          n252 = invoke class="VI" method="Ctrl Val.Get"(reference=w367, "Control Name"="SetVoltageStr") -> (reference out=w361:refnum<vi>, error out=w371:errorcluster, "Get Control Value Variant"=w375:variant)  [unwired: 2 in, 1 out]
          n253 = Variant To Data(error in=w371, type="" ("Control Name"), Variant=w375) -> (data=w370:string, error out=w369:errorcluster)
          n254 = Scan From String(format string="%f", input string=w370, error in=w369) -> (error out=w360:errorcluster, output 1=w358:dbl)  [unwired: 2 in, 2 out]
          n255 = local read "Common volt. inc"() -> (w357:bool)
          n256 = local read "Common volt. dec"() -> (w355:bool)
          n257 = case shown="True" w357 {
            tunnel: "Comm. voltage %" -> [w381 w385]
            tunnel: w358 -> [w382 w384]
            tunnel: [w382 w383] -> w356
            tunnel: [w381 _] -> w354
            frame False {
            }
            frame True {
              n258 = Add(x=w384, y=w385) -> (x+y=w383:dbl)
            }
          }
          n259 = case shown="False" w355 {
            tunnel: w356 -> [w377 w380]
            tunnel: [w377 w379] -> w353
            tunnel: w354 -> [_ w378]
            frame False {
            }
            frame True {
              n260 = Subtract(x=w380, y=w378) -> (x-y=w379:dbl)
            }
          }
          n261 = invoke class="VI" method="Ctrl Val.Set"(reference=w361, error in=w360, "Control Name"="SetVoltage", "Value"=w353) -> (reference out=w363:refnum<vi>, error out=w362:errorcluster)  [unwired: 1 in, 3 out]
          n262 = invoke class="VI" method="Ctrl Val.Set"(reference=w363, error in=w362, "Control Name"="NeedToSetVoltage", "Value"=TRUE ("ConnectChannel")) -> (error out=w359:errorcluster)  [unwired: 1 in, 4 out]
        }
        n263 = Merge Errors(w347) -> (w346:errorcluster)
        n264 = flat-sequence {
          tunnel: w346 -> [w351]
          tunnel: [w351] -> w345
          frame #0 {
            w350 = FALSE ("ConnectChannel")
            n265 = local write "Common volt. inc"(w350) -> ()
            n266 = local write "Common volt. dec"(w350) -> ()
          }
        }
      }
      event "DisconnectChannel": Value Change {
        n267 = event-data() -> ()  [unwired: 7 out]
        n268 = property on="List of channels" class="MCListbox (strict)"() -> ("Value"=w390:i32)  [unwired: 2 in, 2 out]
        n269 = flat-sequence {
          tunnel: w390 -> [w392]
          tunnel: [w392] -> w389
          tunnel: w389 -> [w394]
          tunnel: [w393] -> w387
          tunnel: [w399] -> w388
          tunnel: w387 -> [w399]
          frame #0 {
            w391 = u8 2 ("Disabled")
            n270 = property on="AddChannel" class="Bool (strict)"("Disabled"=w391) -> ()  [unwired: 2 in, 2 out]
            n271 = property on="Set Output ON All" class="Bool (strict)"("Disabled"=w391) -> ()  [unwired: 2 in, 2 out]
            n272 = property on="ConnectAll" class="Bool (strict)"("Disabled"=w391) -> ()  [unwired: 2 in, 2 out]
            n273 = property on="DisconnectChannel" class="Bool (strict)"("Disabled"=w391) -> ()  [unwired: 2 in, 2 out]
            n274 = property on="ReadFromFile" class="Bool (strict)"("Disabled"=w391) -> ()  [unwired: 2 in, 2 out]
            n275 = property on="Quit" class="Bool (strict)"("Disabled"=w391) -> ()  [unwired: 2 in, 2 out]
            n276 = property on="ConnectChannel" class="Bool (strict)"("Disabled"=w391) -> ()  [unwired: 2 in, 2 out]
            n277 = property on="DeleteChannel" class="Bool (strict)"("Disabled"=w391) -> ()  [unwired: 2 in, 2 out]
            n278 = property on="WriteToFile" class="Bool (strict)"("Disabled"=w391) -> ()  [unwired: 2 in, 2 out]
            n279 = property on="SetCurrentB" class="Bool (strict)"("Disabled"=w391) -> ()  [unwired: 2 in, 2 out]
            n280 = property on="SetOutputOnB" class="Bool (strict)"("Disabled"=w391) -> ()  [unwired: 2 in, 2 out]
            n281 = property on="SetVoltageB" class="Bool (strict)"("Disabled"=w391) -> ()  [unwired: 2 in, 2 out]
            n282 = property on="SetOutputOffB" class="Bool (strict)"("Disabled"=w391) -> ()  [unwired: 2 in, 2 out]
            n283 = property on="SetVoltageAll" class="Bool (strict)"("Disabled"=w391) -> ()  [unwired: 2 in, 2 out]
            n284 = property on="SetCurrentAll" class="Bool (strict)"("Disabled"=w391) -> ()  [unwired: 2 in, 2 out]
            n285 = property on="DisconnectAll" class="Bool (strict)"("Disabled"=w391) -> ()  [unwired: 2 in, 2 out]
          }
          frame #1 {
            w395 = FALSE ("OK Button")
            n286 = local write "DisconnectChannel"(w395) -> ()
            n287 = local read "Measure_VI"() -> (w397:refnum<vi>[])
            n288 = Index Array(array=w397, index=w394) -> (element=w396:refnum<vi>)
            n289 = invoke class="VI" method="Ctrl Val.Set"(reference=w396, "Control Name"="Connect", "Value"=w395) -> (error out=w393:errorcluster)  [unwired: 2 in, 4 out]
          }
          frame #2 {
            w400 = u8 0 ("Disabled")
            n290 = property on="AddChannel" class="Bool (strict)"("Disabled"=w400) -> ()  [unwired: 2 in, 2 out]
            n291 = property on="DisconnectChannel" class="Bool (strict)"("Disabled"=w400) -> ()  [unwired: 2 in, 2 out]
            n292 = property on="ConnectAll" class="Bool (strict)"("Disabled"=w400) -> ()  [unwired: 2 in, 2 out]
            n293 = property on="ReadFromFile" class="Bool (strict)"("Disabled"=w400) -> ()  [unwired: 2 in, 2 out]
            n294 = property on="ConnectChannel" class="Bool (strict)"("Disabled"=w400) -> ()  [unwired: 2 in, 2 out]
            n295 = property on="Quit" class="Bool (strict)"("Disabled"=w400) -> ()  [unwired: 2 in, 2 out]
            n296 = property on="DeleteChannel" class="Bool (strict)"("Disabled"=w400) -> ()  [unwired: 2 in, 2 out]
            n297 = property on="SetOutputOffB" class="Bool (strict)"("Disabled"=w400) -> ()  [unwired: 2 in, 2 out]
            n298 = property on="Set Output ON All" class="Bool (strict)"("Disabled"=w400) -> ()  [unwired: 2 in, 2 out]
            n299 = property on="SetVoltageAll" class="Bool (strict)"("Disabled"=w400) -> ()  [unwired: 2 in, 2 out]
            n300 = property on="SetCurrentAll" class="Bool (strict)"("Disabled"=w400) -> ()  [unwired: 2 in, 2 out]
            n301 = property on="DisconnectAll" class="Bool (strict)"("Disabled"=w400) -> ()  [unwired: 2 in, 2 out]
            n302 = property on="WriteToFile" class="Bool (strict)"("Disabled"=w400) -> ()  [unwired: 2 in, 2 out]
            n303 = property on="SetCurrentB" class="Bool (strict)"("Disabled"=w400) -> ()  [unwired: 2 in, 2 out]
            n304 = property on="SetOutputOnB" class="Bool (strict)"("Disabled"=w400) -> ()  [unwired: 2 in, 2 out]
            n305 = property on="SetVoltageB" class="Bool (strict)"("Disabled"=w400) -> ()  [unwired: 2 in, 2 out]
          }
        }
        n306 = Merge Errors(w388) -> (w386:errorcluster)
      }
      event "ConnectChannel": Value Change {
        n307 = event-data() -> ()  [unwired: 7 out]
        n308 = property on="List of channels" class="MCListbox (strict)"() -> ("Value"=w405:i32)  [unwired: 2 in, 2 out]
        n309 = flat-sequence {
          tunnel: w405 -> [w407]
          tunnel: [w407] -> w404
          tunnel: w404 -> [w412]
          tunnel: [w411] -> w402
          tunnel: [w424] -> w403
          tunnel: w402 -> [w424]
          frame #0 {
            w406 = u8 2 ("Disabled")
            n310 = property on="AddChannel" class="Bool (strict)"("Disabled"=w406) -> ()  [unwired: 2 in, 2 out]
            n311 = property on="Set Output ON All" class="Bool (strict)"("Disabled"=w406) -> ()  [unwired: 2 in, 2 out]
            n312 = property on="ConnectAll" class="Bool (strict)"("Disabled"=w406) -> ()  [unwired: 2 in, 2 out]
            n313 = property on="DisconnectChannel" class="Bool (strict)"("Disabled"=w406) -> ()  [unwired: 2 in, 2 out]
            n314 = property on="ReadFromFile" class="Bool (strict)"("Disabled"=w406) -> ()  [unwired: 2 in, 2 out]
            n315 = property on="Quit" class="Bool (strict)"("Disabled"=w406) -> ()  [unwired: 2 in, 2 out]
            n316 = property on="ConnectChannel" class="Bool (strict)"("Disabled"=w406) -> ()  [unwired: 2 in, 2 out]
            n317 = property on="DeleteChannel" class="Bool (strict)"("Disabled"=w406) -> ()  [unwired: 2 in, 2 out]
            n318 = property on="WriteToFile" class="Bool (strict)"("Disabled"=w406) -> ()  [unwired: 2 in, 2 out]
            n319 = property on="SetCurrentB" class="Bool (strict)"("Disabled"=w406) -> ()  [unwired: 2 in, 2 out]
            n320 = property on="SetOutputOnB" class="Bool (strict)"("Disabled"=w406) -> ()  [unwired: 2 in, 2 out]
            n321 = property on="SetVoltageB" class="Bool (strict)"("Disabled"=w406) -> ()  [unwired: 2 in, 2 out]
            n322 = property on="SetOutputOffB" class="Bool (strict)"("Disabled"=w406) -> ()  [unwired: 2 in, 2 out]
            n323 = property on="SetVoltageAll" class="Bool (strict)"("Disabled"=w406) -> ()  [unwired: 2 in, 2 out]
            n324 = property on="SetCurrentAll" class="Bool (strict)"("Disabled"=w406) -> ()  [unwired: 2 in, 2 out]
            n325 = property on="DisconnectAll" class="Bool (strict)"("Disabled"=w406) -> ()  [unwired: 2 in, 2 out]
          }
          frame #1 {
            n326 = local read "Measure_VI"() -> (w413:refnum<vi>[])
            n327 = Index Array(array=w413, index=w412) -> (element=w410:refnum<vi>)
            n328 = flat-sequence {
              tunnel: w410 -> [w415]
              tunnel: [w414] -> w408
              tunnel: [w418] -> w409
              tunnel: w408 -> [w418]
              tunnel: [w420] -> w411
              tunnel: w409 -> [w421]
              frame #0 {
                n329 = invoke class="VI" method="Ctrl Val.Set"(reference=w415, "Control Name"="Connect", "Value"=FALSE ("OK Button")) -> (reference out=w414:refnum<vi>)  [unwired: 2 in, 4 out]
              }
              frame #1 {
                n330 = Wait (ms)(milliseconds to wait=u32 1000) -> ()  [unwired: 1 out]
              }
              frame #2 {
                n331 = invoke class="VI" method="Ctrl Val.Set"(reference=w421, "Control Name"="Connect", "Value"=TRUE ("OK Button")) -> (error out=w420:errorcluster)  [unwired: 2 in, 4 out]
              }
            }
          }
          frame #2 {
            w425 = u8 0 ("Disabled")
            n332 = local write "ConnectChannel"(FALSE ("ConnectChannel")) -> ()
            n333 = property on="ConnectAll" class="Bool (strict)"("Disabled"=w425) -> ()  [unwired: 2 in, 2 out]
            n334 = property on="Set Output ON All" class="Bool (strict)"("Disabled"=w425) -> ()  [unwired: 2 in, 2 out]
            n335 = property on="AddChannel" class="Bool (strict)"("Disabled"=w425) -> ()  [unwired: 2 in, 2 out]
            n336 = property on="DisconnectChannel" class="Bool (strict)"("Disabled"=w425) -> ()  [unwired: 2 in, 2 out]
            n337 = property on="ReadFromFile" class="Bool (strict)"("Disabled"=w425) -> ()  [unwired: 2 in, 2 out]
            n338 = property on="ConnectChannel" class="Bool (strict)"("Disabled"=w425) -> ()  [unwired: 2 in, 2 out]
            n339 = property on="Quit" class="Bool (strict)"("Disabled"=w425) -> ()  [unwired: 2 in, 2 out]
            n340 = property on="DeleteChannel" class="Bool (strict)"("Disabled"=w425) -> ()  [unwired: 2 in, 2 out]
            n341 = property on="WriteToFile" class="Bool (strict)"("Disabled"=w425) -> ()  [unwired: 2 in, 2 out]
            n342 = property on="SetCurrentB" class="Bool (strict)"("Disabled"=w425) -> ()  [unwired: 2 in, 2 out]
            n343 = property on="SetOutputOnB" class="Bool (strict)"("Disabled"=w425) -> ()  [unwired: 2 in, 2 out]
            n344 = property on="SetVoltageB" class="Bool (strict)"("Disabled"=w425) -> ()  [unwired: 2 in, 2 out]
            n345 = property on="SetOutputOffB" class="Bool (strict)"("Disabled"=w425) -> ()  [unwired: 2 in, 2 out]
            n346 = property on="SetVoltageAll" class="Bool (strict)"("Disabled"=w425) -> ()  [unwired: 2 in, 2 out]
            n347 = property on="SetCurrentAll" class="Bool (strict)"("Disabled"=w425) -> ()  [unwired: 2 in, 2 out]
            n348 = property on="DisconnectAll" class="Bool (strict)"("Disabled"=w425) -> ()  [unwired: 2 in, 2 out]
          }
        }
        n349 = Merge Errors(w403) -> (w401:errorcluster)
      }
      event "ConnectAll": Value Change {
        n350 = event-data() -> ()  [unwired: 7 out]
        n351 = flat-sequence {
          tunnel: [w431] -> w428
          tunnel: [w440] -> w429
          tunnel: w428 -> [w440]
          frame #0 {
            w430 = u8 2 ("Disabled")
            n352 = property on="Quit" class="Bool (strict)"("Disabled"=w430) -> ()  [unwired: 2 in, 2 out]
            n353 = property on="ReadFromFile" class="Bool (strict)"("Disabled"=w430) -> ()  [unwired: 2 in, 2 out]
            n354 = property on="WriteToFile" class="Bool (strict)"("Disabled"=w430) -> ()  [unwired: 2 in, 2 out]
            n355 = property on="ConnectAll" class="Bool (strict)"("Disabled"=w430) -> ()  [unwired: 2 in, 2 out]
            n356 = property on="Set Output ON All" class="Bool (strict)"("Disabled"=w430) -> ()  [unwired: 2 in, 2 out]
            n357 = property on="SetOutputOffB" class="Bool (strict)"("Disabled"=w430) -> ()  [unwired: 2 in, 2 out]
            n358 = property on="AddChannel" class="Bool (strict)"("Disabled"=w430) -> ()  [unwired: 2 in, 2 out]
            n359 = property on="DisconnectChannel" class="Bool (strict)"("Disabled"=w430) -> ()  [unwired: 2 in, 2 out]
            n360 = property on="SetCurrentAll" class="Bool (strict)"("Disabled"=w430) -> ()  [unwired: 2 in, 2 out]
            n361 = property on="SetOutputOnB" class="Bool (strict)"("Disabled"=w430) -> ()  [unwired: 2 in, 2 out]
            n362 = property on="ConnectChannel" class="Bool (strict)"("Disabled"=w430) -> ()  [unwired: 2 in, 2 out]
            n363 = property on="DeleteChannel" class="Bool (strict)"("Disabled"=w430) -> ()  [unwired: 2 in, 2 out]
            n364 = property on="SetCurrentB" class="Bool (strict)"("Disabled"=w430) -> ()  [unwired: 2 in, 2 out]
            n365 = property on="SetVoltageB" class="Bool (strict)"("Disabled"=w430) -> ()  [unwired: 2 in, 2 out]
            n366 = property on="SetVoltageAll" class="Bool (strict)"("Disabled"=w430) -> ()  [unwired: 2 in, 2 out]
            n367 = property on="DisconnectAll" class="Bool (strict)"("Disabled"=w430) -> ()  [unwired: 2 in, 2 out]
          }
          frame #1 {
            n368 = local read "Measure_VI"() -> (w433:refnum<vi>[])
            n369 = Array Size(array=w433) -> (size(s)=w432:i32)
            n370 = for {
              N: w432 -> [_]
              tunnel: [w434] -> w431 mode=indexing
              i -> [w435]
              n371 = local read "Measure_VI"() -> (w438:refnum<vi>[])
              n372 = Index Array(array=w438, index=w435) -> (element=w437:refnum<vi>)
              n373 = invoke class="VI" method="Ctrl Val.Set"(reference=w437, "Control Name"="Connect", "Value"=TRUE ("OK Button")) -> (error out=w434:errorcluster)  [unwired: 2 in, 4 out]
            }
          }
          frame #2 {
            w441 = u8 0 ("Disabled")
            n374 = local write "ConnectAll"(FALSE ("ConnectChannel")) -> ()
            n375 = property on="Quit" class="Bool (strict)"("Disabled"=w441) -> ()  [unwired: 2 in, 2 out]
            n376 = property on="AddChannel" class="Bool (strict)"("Disabled"=w441) -> ()  [unwired: 2 in, 2 out]
            n377 = property on="DisconnectChannel" class="Bool (strict)"("Disabled"=w441) -> ()  [unwired: 2 in, 2 out]
            n378 = property on="ConnectAll" class="Bool (strict)"("Disabled"=w441) -> ()  [unwired: 2 in, 2 out]
            n379 = property on="Set Output ON All" class="Bool (strict)"("Disabled"=w441) -> ()  [unwired: 2 in, 2 out]
            n380 = property on="SetOutputOffB" class="Bool (strict)"("Disabled"=w441) -> ()  [unwired: 2 in, 2 out]
            n381 = property on="SetCurrentAll" class="Bool (strict)"("Disabled"=w441) -> ()  [unwired: 2 in, 2 out]
            n382 = property on="ConnectChannel" class="Bool (strict)"("Disabled"=w441) -> ()  [unwired: 2 in, 2 out]
            n383 = property on="SetVoltageAll" class="Bool (strict)"("Disabled"=w441) -> ()  [unwired: 2 in, 2 out]
            n384 = property on="SetOutputOnB" class="Bool (strict)"("Disabled"=w441) -> ()  [unwired: 2 in, 2 out]
            n385 = property on="DisconnectAll" class="Bool (strict)"("Disabled"=w441) -> ()  [unwired: 2 in, 2 out]
            n386 = property on="ReadFromFile" class="Bool (strict)"("Disabled"=w441) -> ()  [unwired: 2 in, 2 out]
            n387 = property on="WriteToFile" class="Bool (strict)"("Disabled"=w441) -> ()  [unwired: 2 in, 2 out]
            n388 = property on="SetCurrentB" class="Bool (strict)"("Disabled"=w441) -> ()  [unwired: 2 in, 2 out]
            n389 = property on="SetVoltageB" class="Bool (strict)"("Disabled"=w441) -> ()  [unwired: 2 in, 2 out]
            n390 = property on="DeleteChannel" class="Bool (strict)"("Disabled"=w441) -> ()  [unwired: 2 in, 2 out]
          }
        }
        n391 = Merge Errors(w429) -> (w427:errorcluster)
      }
      event "DisconnectAll": Value Change {
        n392 = event-data() -> ()  [unwired: 7 out]
        n393 = flat-sequence {
          tunnel: [w447] -> w445
          tunnel: [w456] -> w444
          tunnel: w445 -> [w456]
          frame #0 {
            w446 = u8 2 ("Disabled")
            n394 = property on="Quit" class="Bool (strict)"("Disabled"=w446) -> ()  [unwired: 2 in, 2 out]
            n395 = property on="ReadFromFile" class="Bool (strict)"("Disabled"=w446) -> ()  [unwired: 2 in, 2 out]
            n396 = property on="ConnectAll" class="Bool (strict)"("Disabled"=w446) -> ()  [unwired: 2 in, 2 out]
            n397 = property on="ConnectChannel" class="Bool (strict)"("Disabled"=w446) -> ()  [unwired: 2 in, 2 out]
            n398 = property on="AddChannel" class="Bool (strict)"("Disabled"=w446) -> ()  [unwired: 2 in, 2 out]
            n399 = property on="DisconnectChannel" class="Bool (strict)"("Disabled"=w446) -> ()  [unwired: 2 in, 2 out]
            n400 = property on="Set Output ON All" class="Bool (strict)"("Disabled"=w446) -> ()  [unwired: 2 in, 2 out]
            n401 = property on="WriteToFile" class="Bool (strict)"("Disabled"=w446) -> ()  [unwired: 2 in, 2 out]
            n402 = property on="SetOutputOffB" class="Bool (strict)"("Disabled"=w446) -> ()  [unwired: 2 in, 2 out]
            n403 = property on="SetCurrentAll" class="Bool (strict)"("Disabled"=w446) -> ()  [unwired: 2 in, 2 out]
            n404 = property on="SetOutputOnB" class="Bool (strict)"("Disabled"=w446) -> ()  [unwired: 2 in, 2 out]
            n405 = property on="DeleteChannel" class="Bool (strict)"("Disabled"=w446) -> ()  [unwired: 2 in, 2 out]
            n406 = property on="SetCurrentB" class="Bool (strict)"("Disabled"=w446) -> ()  [unwired: 2 in, 2 out]
            n407 = property on="SetVoltageB" class="Bool (strict)"("Disabled"=w446) -> ()  [unwired: 2 in, 2 out]
            n408 = property on="SetVoltageAll" class="Bool (strict)"("Disabled"=w446) -> ()  [unwired: 2 in, 2 out]
            n409 = property on="DisconnectAll" class="Bool (strict)"("Disabled"=w446) -> ()  [unwired: 2 in, 2 out]
          }
          frame #1 {
            n410 = local read "Measure_VI"() -> (w449:refnum<vi>[])
            n411 = Array Size(array=w449) -> (size(s)=w448:i32)
            n412 = for {
              N: w448 -> [_]
              tunnel: [w450] -> w447 mode=indexing
              i -> [w451]
              n413 = local read "Measure_VI"() -> (w454:refnum<vi>[])
              n414 = Index Array(array=w454, index=w451) -> (element=w453:refnum<vi>)
              n415 = invoke class="VI" method="Ctrl Val.Set"(reference=w453, "Control Name"="Connect", "Value"=FALSE ("OK Button")) -> (error out=w450:errorcluster)  [unwired: 2 in, 4 out]
            }
          }
          frame #2 {
            w457 = u8 0 ("Disabled")
            n416 = local write "DisconnectAll"(FALSE ("ConnectChannel")) -> ()
            n417 = property on="Quit" class="Bool (strict)"("Disabled"=w457) -> ()  [unwired: 2 in, 2 out]
            n418 = property on="ConnectAll" class="Bool (strict)"("Disabled"=w457) -> ()  [unwired: 2 in, 2 out]
            n419 = property on="ConnectChannel" class="Bool (strict)"("Disabled"=w457) -> ()  [unwired: 2 in, 2 out]
            n420 = property on="AddChannel" class="Bool (strict)"("Disabled"=w457) -> ()  [unwired: 2 in, 2 out]
            n421 = property on="DisconnectChannel" class="Bool (strict)"("Disabled"=w457) -> ()  [unwired: 2 in, 2 out]
            n422 = property on="ReadFromFile" class="Bool (strict)"("Disabled"=w457) -> ()  [unwired: 2 in, 2 out]
            n423 = property on="Set Output ON All" class="Bool (strict)"("Disabled"=w457) -> ()  [unwired: 2 in, 2 out]
            n424 = property on="WriteToFile" class="Bool (strict)"("Disabled"=w457) -> ()  [unwired: 2 in, 2 out]
            n425 = property on="SetOutputOnB" class="Bool (strict)"("Disabled"=w457) -> ()  [unwired: 2 in, 2 out]
            n426 = property on="SetCurrentB" class="Bool (strict)"("Disabled"=w457) -> ()  [unwired: 2 in, 2 out]
            n427 = property on="SetVoltageB" class="Bool (strict)"("Disabled"=w457) -> ()  [unwired: 2 in, 2 out]
            n428 = property on="SetVoltageAll" class="Bool (strict)"("Disabled"=w457) -> ()  [unwired: 2 in, 2 out]
            n429 = property on="DisconnectAll" class="Bool (strict)"("Disabled"=w457) -> ()  [unwired: 2 in, 2 out]
            n430 = property on="DeleteChannel" class="Bool (strict)"("Disabled"=w457) -> ()  [unwired: 2 in, 2 out]
            n431 = property on="SetOutputOffB" class="Bool (strict)"("Disabled"=w457) -> ()  [unwired: 2 in, 2 out]
            n432 = property on="SetCurrentAll" class="Bool (strict)"("Disabled"=w457) -> ()  [unwired: 2 in, 2 out]
          }
        }
        n433 = Merge Errors(w444) -> (w443:errorcluster)
      }
      event "SetVoltageB": Value Change {
        n434 = event-data() -> ()  [unwired: 7 out]
        n435 = local write "SetVoltageB"(FALSE ("ConnectChannel")) -> ()
        n436 = flat-sequence {
          tunnel: [w465] -> w461
          tunnel: [w474] -> w460
          tunnel: w461 -> [w474]
          frame #0 {
            w463 = u8 2 ("Disabled")
            n437 = property on="Quit" class="Bool (strict)"("Disabled"=w463) -> ()  [unwired: 2 in, 2 out]
            n438 = property on="AddChannel" class="Bool (strict)"("Disabled"=w463) -> ()  [unwired: 2 in, 2 out]
            n439 = property on="Set Output ON All" class="Bool (strict)"("Disabled"=w463) -> ()  [unwired: 2 in, 2 out]
            n440 = property on="ConnectAll" class="Bool (strict)"("Disabled"=w463) -> ()  [unwired: 2 in, 2 out]
            n441 = property on="DisconnectChannel" class="Bool (strict)"("Disabled"=w463) -> ()  [unwired: 2 in, 2 out]
            n442 = property on="ReadFromFile" class="Bool (strict)"("Disabled"=w463) -> ()  [unwired: 2 in, 2 out]
            n443 = property on="ConnectChannel" class="Bool (strict)"("Disabled"=w463) -> ()  [unwired: 2 in, 2 out]
            n444 = property on="DeleteChannel" class="Bool (strict)"("Disabled"=w463) -> ()  [unwired: 2 in, 2 out]
            n445 = property on="WriteToFile" class="Bool (strict)"("Disabled"=w463) -> ()  [unwired: 2 in, 2 out]
            n446 = property on="SetCurrentB" class="Bool (strict)"("Disabled"=w463) -> ()  [unwired: 2 in, 2 out]
            n447 = property on="SetOutputOnB" class="Bool (strict)"("Disabled"=w463) -> ()  [unwired: 2 in, 2 out]
            n448 = property on="SetVoltageB" class="Bool (strict)"("Disabled"=w463) -> ()  [unwired: 2 in, 2 out]
            n449 = property on="SetOutputOffB" class="Bool (strict)"("Disabled"=w463) -> ()  [unwired: 2 in, 2 out]
            n450 = property on="SetVoltageAll" class="Bool (strict)"("Disabled"=w463) -> ()  [unwired: 2 in, 2 out]
            n451 = property on="SetCurrentAll" class="Bool (strict)"("Disabled"=w463) -> ()  [unwired: 2 in, 2 out]
            n452 = property on="DisconnectAll" class="Bool (strict)"("Disabled"=w463) -> ()  [unwired: 2 in, 2 out]
          }
          frame #1 {
            n453 = property on="List of channels" class="MCListbox (strict)"() -> ("Value"=w464:i32)  [unwired: 2 in, 2 out]
            n454 = local read "Measure_VI"() -> (w472:refnum<vi>[])
            n455 = local read "SetVoltage"() -> (w470:dbl)
            n456 = Index Array(array=w472, index=w464) -> (element=w471:refnum<vi>)
            n457 = invoke class="VI" method="Ctrl Val.Set"(reference=w471, "Control Name"="SetVoltage", "Value"=w470) -> (reference out=w467:refnum<vi>, error out=w466:errorcluster)  [unwired: 2 in, 3 out]
            n458 = invoke class="VI" method="Ctrl Val.Set"(reference=w467, error in=w466, "Control Name"="NeedToSetVoltage", "Value"=TRUE ("ConnectChannel")) -> (error out=w465:errorcluster)  [unwired: 1 in, 4 out]
          }
          frame #2 {
            w475 = u8 0 ("Disabled")
            n459 = property on="Quit" class="Bool (strict)"("Disabled"=w475) -> ()  [unwired: 2 in, 2 out]
            n460 = property on="ConnectAll" class="Bool (strict)"("Disabled"=w475) -> ()  [unwired: 2 in, 2 out]
            n461 = property on="Set Output ON All" class="Bool (strict)"("Disabled"=w475) -> ()  [unwired: 2 in, 2 out]
            n462 = property on="AddChannel" class="Bool (strict)"("Disabled"=w475) -> ()  [unwired: 2 in, 2 out]
            n463 = property on="DisconnectChannel" class="Bool (strict)"("Disabled"=w475) -> ()  [unwired: 2 in, 2 out]
            n464 = property on="ReadFromFile" class="Bool (strict)"("Disabled"=w475) -> ()  [unwired: 2 in, 2 out]
            n465 = property on="ConnectChannel" class="Bool (strict)"("Disabled"=w475) -> ()  [unwired: 2 in, 2 out]
            n466 = property on="DeleteChannel" class="Bool (strict)"("Disabled"=w475) -> ()  [unwired: 2 in, 2 out]
            n467 = property on="SetVoltageAll" class="Bool (strict)"("Disabled"=w475) -> ()  [unwired: 2 in, 2 out]
            n468 = property on="SetCurrentAll" class="Bool (strict)"("Disabled"=w475) -> ()  [unwired: 2 in, 2 out]
            n469 = property on="DisconnectAll" class="Bool (strict)"("Disabled"=w475) -> ()  [unwired: 2 in, 2 out]
            n470 = property on="WriteToFile" class="Bool (strict)"("Disabled"=w475) -> ()  [unwired: 2 in, 2 out]
            n471 = property on="SetCurrentB" class="Bool (strict)"("Disabled"=w475) -> ()  [unwired: 2 in, 2 out]
            n472 = property on="SetOutputOnB" class="Bool (strict)"("Disabled"=w475) -> ()  [unwired: 2 in, 2 out]
            n473 = property on="SetVoltageB" class="Bool (strict)"("Disabled"=w475) -> ()  [unwired: 2 in, 2 out]
            n474 = property on="SetOutputOffB" class="Bool (strict)"("Disabled"=w475) -> ()  [unwired: 2 in, 2 out]
          }
        }
        n475 = Merge Errors(w460) -> (w459:errorcluster)
      }
      event "SetOutputOnB": Value Change {
        n476 = event-data() -> ()  [unwired: 2 out]
        n477 = property on="List of channels" class="MCListbox (strict)"() -> ("Value"=w479:i32)  [unwired: 2 in, 2 out]
        n478 = flat-sequence {
          tunnel: w479 -> [w481]
          tunnel: [w481] -> w478
          tunnel: w478 -> [w488]
          tunnel: [w483] -> w477
          tunnel: [w493] -> w476
          tunnel: w477 -> [w493]
          frame #0 {
            w480 = u8 2 ("Disabled")
            n479 = property on="ConnectAll" class="Bool (strict)"("Disabled"=w480) -> ()  [unwired: 2 in, 2 out]
            n480 = property on="Set Output ON All" class="Bool (strict)"("Disabled"=w480) -> ()  [unwired: 2 in, 2 out]
            n481 = property on="AddChannel" class="Bool (strict)"("Disabled"=w480) -> ()  [unwired: 2 in, 2 out]
            n482 = property on="DisconnectChannel" class="Bool (strict)"("Disabled"=w480) -> ()  [unwired: 2 in, 2 out]
            n483 = property on="ReadFromFile" class="Bool (strict)"("Disabled"=w480) -> ()  [unwired: 2 in, 2 out]
            n484 = property on="Quit" class="Bool (strict)"("Disabled"=w480) -> ()  [unwired: 2 in, 2 out]
            n485 = property on="ConnectChannel" class="Bool (strict)"("Disabled"=w480) -> ()  [unwired: 2 in, 2 out]
            n486 = property on="DeleteChannel" class="Bool (strict)"("Disabled"=w480) -> ()  [unwired: 2 in, 2 out]
            n487 = property on="WriteToFile" class="Bool (strict)"("Disabled"=w480) -> ()  [unwired: 2 in, 2 out]
            n488 = property on="SetCurrentB" class="Bool (strict)"("Disabled"=w480) -> ()  [unwired: 2 in, 2 out]
            n489 = property on="SetOutputOnB" class="Bool (strict)"("Disabled"=w480) -> ()  [unwired: 2 in, 2 out]
            n490 = property on="SetVoltageB" class="Bool (strict)"("Disabled"=w480) -> ()  [unwired: 2 in, 2 out]
            n491 = property on="SetOutputOffB" class="Bool (strict)"("Disabled"=w480) -> ()  [unwired: 2 in, 2 out]
            n492 = property on="SetVoltageAll" class="Bool (strict)"("Disabled"=w480) -> ()  [unwired: 2 in, 2 out]
            n493 = property on="SetCurrentAll" class="Bool (strict)"("Disabled"=w480) -> ()  [unwired: 2 in, 2 out]
            n494 = property on="DisconnectAll" class="Bool (strict)"("Disabled"=w480) -> ()  [unwired: 2 in, 2 out]
          }
          frame #1 {
            n495 = local write "SetOutputOnB"(FALSE ("ConnectChannel")) -> ()
            n496 = local read "Measure_VI"() -> (w491:refnum<vi>[])
            n497 = Index Array(array=w491, index=w488) -> (element=w490:refnum<vi>)
            n498 = invoke class="VI" method="Ctrl Val.Set"(reference=w490, "Control Name"="SetOutput", "Value"=TRUE ("ConnectChannel")) -> (reference out=w485:refnum<vi>, error out=w484:errorcluster)  [unwired: 2 in, 3 out]
            n499 = invoke class="VI" method="Ctrl Val.Set"(reference=w485, error in=w484, "Control Name"="NeedToSetOutput", "Value"=TRUE ("ConnectChannel")) -> (error out=w483:errorcluster)  [unwired: 1 in, 4 out]
          }
          frame #2 {
            w494 = u8 0 ("Disabled")
            n500 = property on="ConnectAll" class="Bool (strict)"("Disabled"=w494) -> ()  [unwired: 2 in, 2 out]
            n501 = property on="Set Output ON All" class="Bool (strict)"("Disabled"=w494) -> ()  [unwired: 2 in, 2 out]
            n502 = property on="AddChannel" class="Bool (strict)"("Disabled"=w494) -> ()  [unwired: 2 in, 2 out]
            n503 = property on="DisconnectChannel" class="Bool (strict)"("Disabled"=w494) -> ()  [unwired: 2 in, 2 out]
            n504 = property on="ReadFromFile" class="Bool (strict)"("Disabled"=w494) -> ()  [unwired: 2 in, 2 out]
            n505 = property on="ConnectChannel" class="Bool (strict)"("Disabled"=w494) -> ()  [unwired: 2 in, 2 out]
            n506 = property on="Quit" class="Bool (strict)"("Disabled"=w494) -> ()  [unwired: 2 in, 2 out]
            n507 = property on="DeleteChannel" class="Bool (strict)"("Disabled"=w494) -> ()  [unwired: 2 in, 2 out]
            n508 = property on="SetOutputOffB" class="Bool (strict)"("Disabled"=w494) -> ()  [unwired: 2 in, 2 out]
            n509 = property on="SetVoltageAll" class="Bool (strict)"("Disabled"=w494) -> ()  [unwired: 2 in, 2 out]
            n510 = property on="SetCurrentAll" class="Bool (strict)"("Disabled"=w494) -> ()  [unwired: 2 in, 2 out]
            n511 = property on="DisconnectAll" class="Bool (strict)"("Disabled"=w494) -> ()  [unwired: 2 in, 2 out]
            n512 = property on="WriteToFile" class="Bool (strict)"("Disabled"=w494) -> ()  [unwired: 2 in, 2 out]
            n513 = property on="SetCurrentB" class="Bool (strict)"("Disabled"=w494) -> ()  [unwired: 2 in, 2 out]
            n514 = property on="SetOutputOnB" class="Bool (strict)"("Disabled"=w494) -> ()  [unwired: 2 in, 2 out]
            n515 = property on="SetVoltageB" class="Bool (strict)"("Disabled"=w494) -> ()  [unwired: 2 in, 2 out]
          }
        }
      }
      event "Set Output ON All": Value Change {
        n516 = event-data() -> ("NewVal"=w495:bool)  [unwired: 1 out]
        n517 = flat-sequence {
          tunnel: [w500] -> w496
          tunnel: w495 -> [w500]
          tunnel: [w505] -> w498
          tunnel: w496 -> [w502]
          tunnel: [w516] -> w499
          tunnel: w498 -> [w516]
          frame #0 {
            w501 = u8 2 ("Disabled")
            n518 = property on="Quit" class="Bool (strict)"("Disabled"=w501) -> ()  [unwired: 2 in, 2 out]
            n519 = property on="AddChannel" class="Bool (strict)"("Disabled"=w501) -> ()  [unwired: 2 in, 2 out]
            n520 = property on="DisconnectChannel" class="Bool (strict)"("Disabled"=w501) -> ()  [unwired: 2 in, 2 out]
            n521 = property on="ConnectAll" class="Bool (strict)"("Disabled"=w501) -> ()  [unwired: 2 in, 2 out]
            n522 = property on="ReadFromFile" class="Bool (strict)"("Disabled"=w501) -> ()  [unwired: 2 in, 2 out]
            n523 = property on="ConnectChannel" class="Bool (strict)"("Disabled"=w501) -> ()  [unwired: 2 in, 2 out]
            n524 = property on="DeleteChannel" class="Bool (strict)"("Disabled"=w501) -> ()  [unwired: 2 in, 2 out]
            n525 = property on="WriteToFile" class="Bool (strict)"("Disabled"=w501) -> ()  [unwired: 2 in, 2 out]
            n526 = property on="SetCurrentB" class="Bool (strict)"("Disabled"=w501) -> ()  [unwired: 2 in, 2 out]
            n527 = property on="SetOutputOnB" class="Bool (strict)"("Disabled"=w501) -> ()  [unwired: 2 in, 2 out]
            n528 = property on="SetVoltageB" class="Bool (strict)"("Disabled"=w501) -> ()  [unwired: 2 in, 2 out]
            n529 = property on="SetOutputOffB" class="Bool (strict)"("Disabled"=w501) -> ()  [unwired: 2 in, 2 out]
            n530 = property on="SetVoltageAll" class="Bool (strict)"("Disabled"=w501) -> ()  [unwired: 2 in, 2 out]
            n531 = property on="SetCurrentAll" class="Bool (strict)"("Disabled"=w501) -> ()  [unwired: 2 in, 2 out]
            n532 = property on="DisconnectAll" class="Bool (strict)"("Disabled"=w501) -> ()  [unwired: 2 in, 2 out]
          }
          frame #1 {
            n533 = local read "Measure_VI"() -> (w504:refnum<vi>[])
            n534 = Array Size(array=w504) -> (size(s)=w503:i32)
            n535 = for {
              N: w503 -> [_]
              tunnel: [w507] -> w505 mode=indexing
              tunnel: w502 -> [w506]
              i -> [w509]
              n536 = local read "Measure_VI"() -> (w514:refnum<vi>[])
              n537 = Index Array(array=w514, index=w509) -> (element=w513:refnum<vi>)
              n538 = invoke class="VI" method="Ctrl Val.Set"(reference=w513, "Control Name"="SetOutput", "Value"=w506) -> (reference out=w510:refnum<vi>, error out=w508:errorcluster)  [unwired: 2 in, 3 out]
              n539 = invoke class="VI" method="Ctrl Val.Set"(reference=w510, error in=w508, "Control Name"="NeedToSetOutput", "Value"=TRUE ("ConnectChannel")) -> (error out=w507:errorcluster)  [unwired: 1 in, 4 out]
            }
          }
          frame #2 {
            w517 = u8 0 ("Disabled")
            n540 = disable-structure shown="Disabled" {
              frame Disabled {
                n541 = local write "Set Output ON All"(FALSE ("ConnectChannel")) -> ()
              }
              frame Enabled {
              }
            }
            n542 = property on="Quit" class="Bool (strict)"("Disabled"=w517) -> ()  [unwired: 2 in, 2 out]
            n543 = property on="ConnectAll" class="Bool (strict)"("Disabled"=w517) -> ()  [unwired: 2 in, 2 out]
            n544 = property on="Set Output ON All" class="Bool (strict)"("Disabled"=w517) -> ()  [unwired: 2 in, 2 out]
            n545 = property on="AddChannel" class="Bool (strict)"("Disabled"=w517) -> ()  [unwired: 2 in, 2 out]
            n546 = property on="DisconnectChannel" class="Bool (strict)"("Disabled"=w517) -> ()  [unwired: 2 in, 2 out]
            n547 = property on="ReadFromFile" class="Bool (strict)"("Disabled"=w517) -> ()  [unwired: 2 in, 2 out]
            n548 = property on="ConnectChannel" class="Bool (strict)"("Disabled"=w517) -> ()  [unwired: 2 in, 2 out]
            n549 = property on="DeleteChannel" class="Bool (strict)"("Disabled"=w517) -> ()  [unwired: 2 in, 2 out]
            n550 = property on="SetVoltageB" class="Bool (strict)"("Disabled"=w517) -> ()  [unwired: 2 in, 2 out]
            n551 = property on="SetOutputOffB" class="Bool (strict)"("Disabled"=w517) -> ()  [unwired: 2 in, 2 out]
            n552 = property on="SetVoltageAll" class="Bool (strict)"("Disabled"=w517) -> ()  [unwired: 2 in, 2 out]
            n553 = property on="SetCurrentAll" class="Bool (strict)"("Disabled"=w517) -> ()  [unwired: 2 in, 2 out]
            n554 = property on="DisconnectAll" class="Bool (strict)"("Disabled"=w517) -> ()  [unwired: 2 in, 2 out]
            n555 = property on="WriteToFile" class="Bool (strict)"("Disabled"=w517) -> ()  [unwired: 2 in, 2 out]
            n556 = property on="SetCurrentB" class="Bool (strict)"("Disabled"=w517) -> ()  [unwired: 2 in, 2 out]
            n557 = property on="SetOutputOnB" class="Bool (strict)"("Disabled"=w517) -> ()  [unwired: 2 in, 2 out]
          }
        }
        n558 = Merge Errors(w499) -> (w497:errorcluster)
      }
      event "SetOutputOffB": Value Change {
        n559 = event-data() -> ()  [unwired: 7 out]
        n560 = local write "SetOutputOffB"(FALSE ("ConnectChannel")) -> ()
        n561 = property on="List of channels" class="MCListbox (strict)"() -> ("Value"=w523:i32)  [unwired: 2 in, 2 out]
        n562 = flat-sequence {
          tunnel: w523 -> [w525]
          tunnel: [w525] -> w522
          tunnel: w522 -> [w532]
          tunnel: [w526] -> w519
          tunnel: [w536] -> w520
          tunnel: w519 -> [w536]
          frame #0 {
            w524 = u8 2 ("Disabled")
            n563 = property on="ConnectAll" class="Bool (strict)"("Disabled"=w524) -> ()  [unwired: 2 in, 2 out]
            n564 = property on="Set Output ON All" class="Bool (strict)"("Disabled"=w524) -> ()  [unwired: 2 in, 2 out]
            n565 = property on="AddChannel" class="Bool (strict)"("Disabled"=w524) -> ()  [unwired: 2 in, 2 out]
            n566 = property on="DisconnectChannel" class="Bool (strict)"("Disabled"=w524) -> ()  [unwired: 2 in, 2 out]
            n567 = property on="ReadFromFile" class="Bool (strict)"("Disabled"=w524) -> ()  [unwired: 2 in, 2 out]
            n568 = property on="Quit" class="Bool (strict)"("Disabled"=w524) -> ()  [unwired: 2 in, 2 out]
            n569 = property on="ConnectChannel" class="Bool (strict)"("Disabled"=w524) -> ()  [unwired: 2 in, 2 out]
            n570 = property on="DeleteChannel" class="Bool (strict)"("Disabled"=w524) -> ()  [unwired: 2 in, 2 out]
            n571 = property on="WriteToFile" class="Bool (strict)"("Disabled"=w524) -> ()  [unwired: 2 in, 2 out]
            n572 = property on="SetCurrentB" class="Bool (strict)"("Disabled"=w524) -> ()  [unwired: 2 in, 2 out]
            n573 = property on="SetOutputOnB" class="Bool (strict)"("Disabled"=w524) -> ()  [unwired: 2 in, 2 out]
            n574 = property on="SetVoltageB" class="Bool (strict)"("Disabled"=w524) -> ()  [unwired: 2 in, 2 out]
            n575 = property on="SetOutputOffB" class="Bool (strict)"("Disabled"=w524) -> ()  [unwired: 2 in, 2 out]
            n576 = property on="SetVoltageAll" class="Bool (strict)"("Disabled"=w524) -> ()  [unwired: 2 in, 2 out]
            n577 = property on="SetCurrentAll" class="Bool (strict)"("Disabled"=w524) -> ()  [unwired: 2 in, 2 out]
            n578 = property on="DisconnectAll" class="Bool (strict)"("Disabled"=w524) -> ()  [unwired: 2 in, 2 out]
          }
          frame #1 {
            n579 = local read "Measure_VI"() -> (w534:refnum<vi>[])
            n580 = Index Array(array=w534, index=w532) -> (element=w533:refnum<vi>)
            n581 = invoke class="VI" method="Ctrl Val.Set"(reference=w533, "Control Name"="SetOutput", "Value"=FALSE ("ConnectChannel")) -> (reference out=w529:refnum<vi>, error out=w527:errorcluster)  [unwired: 2 in, 3 out]
            n582 = invoke class="VI" method="Ctrl Val.Set"(reference=w529, error in=w527, "Control Name"="NeedToSetOutput", "Value"=TRUE ("ConnectChannel")) -> (error out=w526:errorcluster)  [unwired: 1 in, 4 out]
          }
          frame #2 {
            w537 = u8 0 ("Disabled")
            n583 = property on="ConnectAll" class="Bool (strict)"("Disabled"=w537) -> ()  [unwired: 2 in, 2 out]
            n584 = property on="Set Output ON All" class="Bool (strict)"("Disabled"=w537) -> ()  [unwired: 2 in, 2 out]
            n585 = property on="AddChannel" class="Bool (strict)"("Disabled"=w537) -> ()  [unwired: 2 in, 2 out]
            n586 = property on="DisconnectChannel" class="Bool (strict)"("Disabled"=w537) -> ()  [unwired: 2 in, 2 out]
            n587 = property on="ReadFromFile" class="Bool (strict)"("Disabled"=w537) -> ()  [unwired: 2 in, 2 out]
            n588 = property on="ConnectChannel" class="Bool (strict)"("Disabled"=w537) -> ()  [unwired: 2 in, 2 out]
            n589 = property on="Quit" class="Bool (strict)"("Disabled"=w537) -> ()  [unwired: 2 in, 2 out]
            n590 = property on="DeleteChannel" class="Bool (strict)"("Disabled"=w537) -> ()  [unwired: 2 in, 2 out]
            n591 = property on="SetOutputOffB" class="Bool (strict)"("Disabled"=w537) -> ()  [unwired: 2 in, 2 out]
            n592 = property on="SetVoltageAll" class="Bool (strict)"("Disabled"=w537) -> ()  [unwired: 2 in, 2 out]
            n593 = property on="SetCurrentAll" class="Bool (strict)"("Disabled"=w537) -> ()  [unwired: 2 in, 2 out]
            n594 = property on="DisconnectAll" class="Bool (strict)"("Disabled"=w537) -> ()  [unwired: 2 in, 2 out]
            n595 = property on="WriteToFile" class="Bool (strict)"("Disabled"=w537) -> ()  [unwired: 2 in, 2 out]
            n596 = property on="SetCurrentB" class="Bool (strict)"("Disabled"=w537) -> ()  [unwired: 2 in, 2 out]
            n597 = property on="SetOutputOnB" class="Bool (strict)"("Disabled"=w537) -> ()  [unwired: 2 in, 2 out]
            n598 = property on="SetVoltageB" class="Bool (strict)"("Disabled"=w537) -> ()  [unwired: 2 in, 2 out]
          }
        }
      }
      event "WriteToFile": Value Change {
        n599 = event-data() -> ()  [unwired: 7 out]
        n600 = local read "ADRESS"() -> (w542:string[])
        n601 = Array Size(array=w542) -> (size(s)=w541:i32)
        n602 = flat-sequence {
          tunnel: w541 -> [w551]
          tunnel: [w543] -> w539
          tunnel: [w584] -> w540
          tunnel: w539 -> [w584]
          frame #0 {
            n603 = Number To Decimal String(number=w551) -> (decimal integer string=w546:string)  [unwired: 1 out]
            n604 = Write to Text File(text=w546) -> (refnum out=w545:refnum<file>, cancelled=w544:bool, error out=w547:errorcluster)  [unwired: 1 in, 2 out]
            n605 = Write to Text File(file (use dialog)=w545, text="\nИМЯ  АДРЕС  ТОК  НАПРЯЖЕНИЕ", error in=w547) -> (refnum out=w548:refnum<file>, error out=w549:errorcluster)  [unwired: 2 out]
            n606 = for {
              N: w551 -> [_]
              tunnel: w544 -> [w561]
              tunnel: w549 -> [w556]
              tunnel: w548 -> [w563]
              tunnel: [w554] -> w543 mode=indexing
              i -> [w562]
              w567 = "" ("Control Name")
              w573 = "\t"
              n607 = local read "Measure_VI"() -> (w571:refnum<vi>[])
              n608 = Index Array(array=w571, index=w562) -> (element=w570:refnum<vi>)
              n609 = invoke class="VI" method="Ctrl Val.Get"(reference=w570, "Control Name"="SetVoltageStr") -> (reference out=w565:refnum<vi>, error out=w558:errorcluster, "Get Control Value Variant"=w572:variant)  [unwired: 2 in, 1 out]
              n610 = invoke class="VI" method="Ctrl Val.Get"(reference=w565, error in=w558, "Control Name"="SetCurrentStr") -> (error out=w557:errorcluster, "Get Control Value Variant"=w568:variant)  [unwired: 1 in, 2 out]
              n611 = local read "ADRESS"() -> (w578:string[])
              n612 = local read "NAME"() -> (w576:string[])
              n613 = Index Array(array=w576, index=w562) -> (element=w574:string)
              n614 = Index Array(array=w578, index=w562) -> (element=w577:string)
              n615 = Variant To Data(type=w567, Variant=w568) -> (data=w552:string, error out=w560:errorcluster)  [unwired: 1 in]
              n616 = Variant To Data(type=w567, Variant=w572) -> (data=w553:string, error out=w559:errorcluster)  [unwired: 1 in]
              n617 = Merge Errors(w557, w560, w559, w556) -> (w555:errorcluster)
              n618 = Concatenate Strings("\r\n", w574, w573, w577, w573, w553, w573, w552) -> (w564:string)
              n619 = case shown="False" w561 {
                tunnel: w563 -> [w581 _]
                tunnel: w564 -> [w582 _]
                tunnel: w555 -> [w580 w583]
                tunnel: [w579 w583] -> w554
                frame False {
                  n620 = Write to Text File(file (use dialog)=w581, text=w582, error in=w580) -> (error out=w579:errorcluster)  [unwired: 3 out]
                }
                frame True {
                }
              }
            }
          }
          frame #1 {
            n621 = local write "WriteToFile"(FALSE ("ConnectChannel")) -> ()
          }
        }
        n622 = Merge Errors(w540) -> (w538:errorcluster)
      }
      event "ReadFromFile": Value Change {
        n623 = event-data() -> ()  [unwired: 2 out]
        n624 = Read from Text File(count=100) -> (text=w592:string[], cancelled=w591:bool, error out=w590:errorcluster)  [unwired: 1 in, 3 out]
        n625 = local read "ReadFromFile"() -> (w588:bool)
        n626 = Not(x=w591) -> (.not. x?=w587:bool)
        n627 = And(x=w588, y=w587) -> (x .and. y?=w586:bool)
        n628 = case shown="True" w586 {
          tunnel: w592 -> [_ w596]
          tunnel: w590 -> [w594 w598]
          tunnel: [w594 w597] -> w589
          frame False {
            n629 = local write "ReadFromFile"(FALSE ("ConnectChannel")) -> ()
          }
          frame True {
            n630 = flat-sequence {
              tunnel: w598 -> [w605]
              tunnel: [w604] -> w600
              tunnel: w600 -> [w619]
              tunnel: [w619] -> w599
              tunnel: w599 -> [_]
              tunnel: [w628] -> w602
              tunnel: w596 -> [w630]
              tunnel: w602 -> [w664]
              tunnel: [w664] -> w601
              frame #0 {
                w603 = u8 2 ("Disabled")
                n631 = disable-structure shown="Enabled" {
                  disable-tunnel: w605 -> [w608 w617]
                  disable-tunnel: [w607 w617] -> w604
                  frame Disabled {
                    n632 = local read "Measure_VI"() -> (w609:refnum<vi>[])
                    n633 = Array Size(array=w609) -> (size(s)=w606:i32)
                    n634 = for {
                      N: w606 -> [_]
                      tunnel: w609 -> [w613]
                      tunnel: w608 -> [w611]
                      tunnel: [w610] -> w607 mode=indexing
                      i -> [w614]
                      n635 = Index Array(array=w613, index=w614) -> (element=w612:refnum<vi>)
                      n636 = invoke class="VI" method="Ctrl Val.Set"(reference=w612, error in=w611, "Control Name"="Connect", "Value"=FALSE) -> (error out=w610:errorcluster)  [unwired: 1 in, 4 out]
                    }
                  }
                  frame Enabled {
                  }
                }
                n637 = property on="Set Output ON All" class="Bool (strict)"("Disabled"=w603) -> ()  [unwired: 2 in, 2 out]
                n638 = property on="ConnectAll" class="Bool (strict)"("Disabled"=w603) -> ()  [unwired: 2 in, 2 out]
                n639 = property on="ReadFromFile" class="Bool (strict)"("Disabled"=w603) -> ()  [unwired: 2 in, 2 out]
                n640 = property on="ConnectChannel" class="Bool (strict)"("Disabled"=w603) -> ()  [unwired: 2 in, 2 out]
                n641 = property on="DisconnectChannel" class="Bool (strict)"("Disabled"=w603) -> ()  [unwired: 2 in, 2 out]
                n642 = property on="WriteToFile" class="Bool (strict)"("Disabled"=w603) -> ()  [unwired: 2 in, 2 out]
                n643 = property on="AddChannel" class="Bool (strict)"("Disabled"=w603) -> ()  [unwired: 2 in, 2 out]
                n644 = property on="SetOutputOnB" class="Bool (strict)"("Disabled"=w603) -> ()  [unwired: 2 in, 2 out]
                n645 = property on="Quit" class="Bool (strict)"("Disabled"=w603) -> ()  [unwired: 2 in, 2 out]
                n646 = property on="DeleteChannel" class="Bool (strict)"("Disabled"=w603) -> ()  [unwired: 2 in, 2 out]
                n647 = property on="SetCurrentB" class="Bool (strict)"("Disabled"=w603) -> ()  [unwired: 2 in, 2 out]
                n648 = property on="SetOutputOffB" class="Bool (strict)"("Disabled"=w603) -> ()  [unwired: 2 in, 2 out]
                n649 = property on="SetCurrentAll" class="Bool (strict)"("Disabled"=w603) -> ()  [unwired: 2 in, 2 out]
                n650 = property on="SetVoltageB" class="Bool (strict)"("Disabled"=w603) -> ()  [unwired: 2 in, 2 out]
                n651 = property on="SetVoltageAll" class="Bool (strict)"("Disabled"=w603) -> ()  [unwired: 2 in, 2 out]
                n652 = property on="DisconnectAll" class="Bool (strict)"("Disabled"=w603) -> ()  [unwired: 2 in, 2 out]
              }
              frame #1 {
                n653 = Wait (ms)(milliseconds to wait=u32 1000) -> ()  [unwired: 1 out]
              }
              frame #2 {
                n654 = local read "Measure_VI"() -> (w622:refnum<vi>[])
                n655 = Wait (ms)(milliseconds to wait=u32 250) -> ()  [unwired: 1 out]
                n656 = Array Size(array=w622) -> (size(s)=w621:i32)
                n657 = for {
                  N: w621 -> [_]
                  tunnel: w622 -> [w624]
                  i -> [w625]
                  n658 = Index Array(array=w624, index=w625) -> (element=w623:refnum<vi>)
                  n659 = invoke class="VI" method="Abort VI"(reference=w623) -> ()  [unwired: 2 in, 3 out]
                }
              }
              frame #3 {
                w627 = string[] [] ("GlobalInAdress")
                n660 = local write "NAME"(w627) -> ()
                n661 = local write "ADRESS"(w627) -> ()
                n662 = local write "Measure_VI"(refnum<vi>[] []) -> ()
              }
              frame #4 {
                n663 = Index Array(array=w630, index=0) -> (element=w633:string)
                n664 = Decimal String To Number(string=w633) -> (number=w631:i32)  [unwired: 3 out]
                n665 = for {
                  N: w631 -> [_]
                  tunnel: w630 -> [w658]
                  tunnel: [w636] -> w629 mode=indexing
                  i -> [w661]
                  n666 = Add(x=2, y=w661) -> (x+y=w660:i32)
                  n667 = Index Array(array=w658, index=w660) -> (element=w657:string)
                  n668 = Spreadsheet String To Array(format string="%s", spreadsheet string=w657, array type (2D Dbl)=string[] [] ("GlobalInAdress")) -> (array=w648:string[])  [unwired: 1 out]
                  n669 = Index Array(array=w648, index=3) -> (element=w634:string)
                  n670 = Index Array(array=w648, index=0) -> (element=w652:string)
                  n671 = Index Array(array=w648, index=1) -> (element=w653:string)
                  n672 = Index Array(array=w648, index=2) -> (element=w635:string)
                  n673 = local read "Measure_VI"() -> (w645:refnum<vi>[])
                  n674 = local read "ADRESS"() -> (w646:string[])
                  n675 = Scan From String(input string=w634, default 1=0.0 ("default value 1")) -> (output 1=w641:dbl)  [unwired: 3 in, 3 out]
                  n676 = Scan From String(input string=w635, default 1=0.0 ("default value 1")) -> (output 1=w643:dbl)  [unwired: 3 in, 3 out]
                  n677 = local read "NAME"() -> (w647:string[])
                  n678 = call "AddChannel.vi"("VIRef"=w645, "Name"=w652, "SetCurrent"=w641, "ADRESS"=w646, "NAME"=w647, "Address"=w653, "SetVoltage"=w643) -> ("NAMEOut"=w640:string[], "error out"=w637:errorcluster, "ADRESSOut"=w638:string[], "VIRefOut"=w639:refnum<vi>[])  [unwired: 1 in, 4 out]
                  n679 = local write "NAME"(w640) -> ()
                  n680 = flat-sequence {
                    tunnel: w637 -> [w663]
                    tunnel: [w663] -> w636
                    frame #0 {
                      n681 = Wait (ms)(milliseconds to wait=u32 50) -> ()  [unwired: 1 out]
                    }
                  }
                  n682 = local write "ADRESS"(w638) -> ()
                  n683 = local write "Measure_VI"(w639) -> ()
                }
                n684 = Merge Errors(w629) -> (w628:errorcluster)
              }
              frame #5 {
                w665 = u8 0 ("Disabled")
                n685 = local write "ReadFromFile"(FALSE ("ConnectChannel")) -> ()
                n686 = property on="ConnectAll" class="Bool (strict)"("Disabled"=w665) -> ()  [unwired: 2 in, 2 out]
                n687 = property on="Set Output ON All" class="Bool (strict)"("Disabled"=w665) -> ()  [unwired: 2 in, 2 out]
                n688 = property on="AddChannel" class="Bool (strict)"("Disabled"=w665) -> ()  [unwired: 2 in, 2 out]
                n689 = property on="DisconnectChannel" class="Bool (strict)"("Disabled"=w665) -> ()  [unwired: 2 in, 2 out]
                n690 = property on="ReadFromFile" class="Bool (strict)"("Disabled"=w665) -> ()  [unwired: 2 in, 2 out]
                n691 = property on="ConnectChannel" class="Bool (strict)"("Disabled"=w665) -> ()  [unwired: 2 in, 2 out]
                n692 = property on="DeleteChannel" class="Bool (strict)"("Disabled"=w665) -> ()  [unwired: 2 in, 2 out]
                n693 = property on="WriteToFile" class="Bool (strict)"("Disabled"=w665) -> ()  [unwired: 2 in, 2 out]
                n694 = property on="SetCurrentB" class="Bool (strict)"("Disabled"=w665) -> ()  [unwired: 2 in, 2 out]
                n695 = property on="Quit" class="Bool (strict)"("Disabled"=w665) -> ()  [unwired: 2 in, 2 out]
                n696 = property on="SetOutputOnB" class="Bool (strict)"("Disabled"=w665) -> ()  [unwired: 2 in, 2 out]
                n697 = property on="SetVoltageB" class="Bool (strict)"("Disabled"=w665) -> ()  [unwired: 2 in, 2 out]
                n698 = property on="SetOutputOffB" class="Bool (strict)"("Disabled"=w665) -> ()  [unwired: 2 in, 2 out]
                n699 = property on="SetVoltageAll" class="Bool (strict)"("Disabled"=w665) -> ()  [unwired: 2 in, 2 out]
                n700 = property on="SetCurrentAll" class="Bool (strict)"("Disabled"=w665) -> ()  [unwired: 2 in, 2 out]
                n701 = property on="DisconnectAll" class="Bool (strict)"("Disabled"=w665) -> ()  [unwired: 2 in, 2 out]
              }
            }
            n702 = Merge Errors(w601) -> (w597:errorcluster)
          }
        }
      }
      event "SetCurrentB": Value Change {
        n703 = event-data() -> ()  [unwired: 7 out]
        n704 = local write "SetCurrentB"(FALSE ("ConnectChannel")) -> ()
        n705 = property on="List of channels" class="MCListbox (strict)"() -> (error out=w669:errorcluster, "Value"=w673:i32)  [unwired: 2 in, 1 out]
        n706 = flat-sequence {
          tunnel: w673 -> [w676]
          tunnel: [w676] -> w672
          tunnel: [w674] -> w670
          tunnel: w669 -> [w674]
          tunnel: w672 -> [w678]
          tunnel: w670 -> [w677]
          tunnel: [w679] -> w668
          tunnel: [w688] -> w667
          tunnel: w668 -> [w688]
          frame #0 {
            w675 = u8 2 ("Disabled")
            n707 = property on="AddChannel" class="Bool (strict)"("Disabled"=w675) -> ()  [unwired: 2 in, 2 out]
            n708 = property on="Set Output ON All" class="Bool (strict)"("Disabled"=w675) -> ()  [unwired: 2 in, 2 out]
            n709 = property on="ConnectAll" class="Bool (strict)"("Disabled"=w675) -> ()  [unwired: 2 in, 2 out]
            n710 = property on="DisconnectChannel" class="Bool (strict)"("Disabled"=w675) -> ()  [unwired: 2 in, 2 out]
            n711 = property on="ReadFromFile" class="Bool (strict)"("Disabled"=w675) -> ()  [unwired: 2 in, 2 out]
            n712 = property on="Quit" class="Bool (strict)"("Disabled"=w675) -> ()  [unwired: 2 in, 2 out]
            n713 = property on="ConnectChannel" class="Bool (strict)"("Disabled"=w675) -> ()  [unwired: 2 in, 2 out]
            n714 = property on="DeleteChannel" class="Bool (strict)"("Disabled"=w675) -> ()  [unwired: 2 in, 2 out]
            n715 = property on="WriteToFile" class="Bool (strict)"("Disabled"=w675) -> ()  [unwired: 2 in, 2 out]
            n716 = property on="SetCurrentB" class="Bool (strict)"("Disabled"=w675) -> ()  [unwired: 2 in, 2 out]
            n717 = property on="SetOutputOnB" class="Bool (strict)"("Disabled"=w675) -> ()  [unwired: 2 in, 2 out]
            n718 = property on="SetVoltageB" class="Bool (strict)"("Disabled"=w675) -> ()  [unwired: 2 in, 2 out]
            n719 = property on="SetOutputOffB" class="Bool (strict)"("Disabled"=w675) -> ()  [unwired: 2 in, 2 out]
            n720 = property on="SetVoltageAll" class="Bool (strict)"("Disabled"=w675) -> ()  [unwired: 2 in, 2 out]
            n721 = property on="SetCurrentAll" class="Bool (strict)"("Disabled"=w675) -> ()  [unwired: 2 in, 2 out]
            n722 = property on="DisconnectAll" class="Bool (strict)"("Disabled"=w675) -> ()  [unwired: 2 in, 2 out]
          }
          frame #1 {
            n723 = local read "Measure_VI"() -> (w686:refnum<vi>[])
            n724 = local read "SetCurrent"() -> (w684:dbl)
            n725 = Index Array(array=w686, index=w678) -> (element=w685:refnum<vi>)
            n726 = invoke class="VI" method="Ctrl Val.Set"(reference=w685, error in=w677, "Control Name"="SetCurrent", "Value"=w684) -> (reference out=w681:refnum<vi>, error out=w680:errorcluster)  [unwired: 1 in, 3 out]
            n727 = invoke class="VI" method="Ctrl Val.Set"(reference=w681, error in=w680, "Control Name"="NeedToSetCurrent", "Value"=TRUE ("ConnectChannel")) -> (error out=w679:errorcluster)  [unwired: 1 in, 4 out]
          }
          frame #2 {
            w689 = u8 0 ("Disabled")
            n728 = property on="AddChannel" class="Bool (strict)"("Disabled"=w689) -> ()  [unwired: 2 in, 2 out]
            n729 = property on="Set Output ON All" class="Bool (strict)"("Disabled"=w689) -> ()  [unwired: 2 in, 2 out]
            n730 = property on="DisconnectChannel" class="Bool (strict)"("Disabled"=w689) -> ()  [unwired: 2 in, 2 out]
            n731 = property on="ConnectAll" class="Bool (strict)"("Disabled"=w689) -> ()  [unwired: 2 in, 2 out]
            n732 = property on="ReadFromFile" class="Bool (strict)"("Disabled"=w689) -> ()  [unwired: 2 in, 2 out]
            n733 = property on="ConnectChannel" class="Bool (strict)"("Disabled"=w689) -> ()  [unwired: 2 in, 2 out]
            n734 = property on="DeleteChannel" class="Bool (strict)"("Disabled"=w689) -> ()  [unwired: 2 in, 2 out]
            n735 = property on="Quit" class="Bool (strict)"("Disabled"=w689) -> ()  [unwired: 2 in, 2 out]
            n736 = property on="WriteToFile" class="Bool (strict)"("Disabled"=w689) -> ()  [unwired: 2 in, 2 out]
            n737 = property on="SetCurrentB" class="Bool (strict)"("Disabled"=w689) -> ()  [unwired: 2 in, 2 out]
            n738 = property on="SetOutputOnB" class="Bool (strict)"("Disabled"=w689) -> ()  [unwired: 2 in, 2 out]
            n739 = property on="SetVoltageB" class="Bool (strict)"("Disabled"=w689) -> ()  [unwired: 2 in, 2 out]
            n740 = property on="SetOutputOffB" class="Bool (strict)"("Disabled"=w689) -> ()  [unwired: 2 in, 2 out]
            n741 = property on="SetVoltageAll" class="Bool (strict)"("Disabled"=w689) -> ()  [unwired: 2 in, 2 out]
            n742 = property on="SetCurrentAll" class="Bool (strict)"("Disabled"=w689) -> ()  [unwired: 2 in, 2 out]
            n743 = property on="DisconnectAll" class="Bool (strict)"("Disabled"=w689) -> ()  [unwired: 2 in, 2 out]
          }
        }
      }
      event "DeleteChannel": Value Change {
        n744 = event-data() -> ()  [unwired: 7 out]
        n745 = property on="List of channels" class="MCListbox (strict)"() -> ("Value"=w693:i32)  [unwired: 2 in, 2 out]
        n746 = flat-sequence {
          tunnel: [w702] -> w694
          tunnel: w693 -> [w702]
          tunnel: [w706] -> w701
          tunnel: [w704] -> w700
          tunnel: [w705] -> w699
          tunnel: w694 -> [w704]
          tunnel: [w712] -> w698
          tunnel: w701 -> [w712]
          tunnel: [w711] -> w697
          tunnel: w700 -> [w711]
          tunnel: w699 -> [w710]
          tunnel: [w710] -> w696
          tunnel: w698 -> [w717]
          tunnel: [w716] -> w695
          tunnel: w697 -> [w716]
          tunnel: w696 -> [w715]
          tunnel: [w714] -> w691
          tunnel: w695 -> [w719]
          tunnel: [w718] -> w692
          tunnel: w691 -> [w718]
          tunnel: w692 -> [w727]
          tunnel: [w727] -> w690
          frame #0 {
            w703 = u8 2 ("Disabled")
            n747 = property on="AddChannel" class="Bool (strict)"("Disabled"=w703) -> ()  [unwired: 2 in, 2 out]
            n748 = property on="Set Output ON All" class="Bool (strict)"("Disabled"=w703) -> ()  [unwired: 2 in, 2 out]
            n749 = property on="ConnectAll" class="Bool (strict)"("Disabled"=w703) -> ()  [unwired: 2 in, 2 out]
            n750 = property on="DisconnectChannel" class="Bool (strict)"("Disabled"=w703) -> ()  [unwired: 2 in, 2 out]
            n751 = property on="ReadFromFile" class="Bool (strict)"("Disabled"=w703) -> ()  [unwired: 2 in, 2 out]
            n752 = property on="Quit" class="Bool (strict)"("Disabled"=w703) -> ()  [unwired: 2 in, 2 out]
            n753 = property on="ConnectChannel" class="Bool (strict)"("Disabled"=w703) -> ()  [unwired: 2 in, 2 out]
            n754 = property on="DeleteChannel" class="Bool (strict)"("Disabled"=w703) -> ()  [unwired: 2 in, 2 out]
            n755 = property on="WriteToFile" class="Bool (strict)"("Disabled"=w703) -> ()  [unwired: 2 in, 2 out]
            n756 = property on="SetCurrentB" class="Bool (strict)"("Disabled"=w703) -> ()  [unwired: 2 in, 2 out]
            n757 = property on="SetOutputOnB" class="Bool (strict)"("Disabled"=w703) -> ()  [unwired: 2 in, 2 out]
            n758 = property on="SetVoltageB" class="Bool (strict)"("Disabled"=w703) -> ()  [unwired: 2 in, 2 out]
            n759 = property on="SetOutputOffB" class="Bool (strict)"("Disabled"=w703) -> ()  [unwired: 2 in, 2 out]
            n760 = property on="SetVoltageAll" class="Bool (strict)"("Disabled"=w703) -> ()  [unwired: 2 in, 2 out]
            n761 = property on="SetCurrentAll" class="Bool (strict)"("Disabled"=w703) -> ()  [unwired: 2 in, 2 out]
            n762 = property on="DisconnectAll" class="Bool (strict)"("Disabled"=w703) -> ()  [unwired: 2 in, 2 out]
          }
          frame #1 {
            n763 = local read "Measure_VI"() -> (w708:refnum<vi>[])
            n764 = Index Array(array=w708, index=w704) -> (element=w706:refnum<vi>)
            n765 = invoke class="VI" method="Ctrl Val.Set"(reference=w706, "Control Name"="Connect", "Value"=FALSE ("OK Button")) -> (error out=w705:errorcluster)  [unwired: 2 in, 4 out]
          }
          frame #2 {
            n766 = Wait (ms)(milliseconds to wait=u32 1000) -> ()  [unwired: 1 out]
          }
          frame #3 {
            n767 = invoke class="VI" method="Abort VI"(reference=w717, error in=w715) -> (error out=w714:errorcluster)  [unwired: 1 in, 2 out]
          }
          frame #4 {
            w720 = 1 ("length")
            n768 = local read "Measure_VI"() -> (w726:refnum<vi>[])
            n769 = local read "ADRESS"() -> (w725:string[])
            n770 = local read "NAME"() -> (w721:string[])
            n771 = Delete From Array(array=w726, length=w720, index=w719) -> (array with subset deleted=w723:refnum<vi>[])  [unwired: 1 out]
            n772 = Delete From Array(array=w725, length=w720, index=w719) -> (array with subset deleted=w724:string[])  [unwired: 1 out]
            n773 = Delete From Array(array=w721, length=w720, index=w719) -> (array with subset deleted=w722:string[])  [unwired: 1 out]
            n774 = local write "ADRESS"(w724) -> ()
            n775 = local write "Measure_VI"(w723) -> ()
            n776 = local write "NAME"(w722) -> ()
          }
          frame #5 {
            w728 = u8 0 ("Disabled")
            n777 = local write "DeleteChannel"(FALSE ("DeleteChannel")) -> ()
            n778 = property on="AddChannel" class="Bool (strict)"("Disabled"=w728) -> ()  [unwired: 2 in, 2 out]
            n779 = property on="DisconnectChannel" class="Bool (strict)"("Disabled"=w728) -> ()  [unwired: 2 in, 2 out]
            n780 = property on="ReadFromFile" class="Bool (strict)"("Disabled"=w728) -> ()  [unwired: 2 in, 2 out]
            n781 = property on="ConnectChannel" class="Bool (strict)"("Disabled"=w728) -> ()  [unwired: 2 in, 2 out]
            n782 = property on="Quit" class="Bool (strict)"("Disabled"=w728) -> ()  [unwired: 2 in, 2 out]
            n783 = property on="DeleteChannel" class="Bool (strict)"("Disabled"=w728) -> ()  [unwired: 2 in, 2 out]
            n784 = property on="WriteToFile" class="Bool (strict)"("Disabled"=w728) -> ()  [unwired: 2 in, 2 out]
            n785 = property on="Set Output ON All" class="Bool (strict)"("Disabled"=w728) -> ()  [unwired: 2 in, 2 out]
            n786 = property on="SetCurrentB" class="Bool (strict)"("Disabled"=w728) -> ()  [unwired: 2 in, 2 out]
            n787 = property on="ConnectAll" class="Bool (strict)"("Disabled"=w728) -> ()  [unwired: 2 in, 2 out]
            n788 = property on="SetOutputOnB" class="Bool (strict)"("Disabled"=w728) -> ()  [unwired: 2 in, 2 out]
            n789 = property on="SetVoltageB" class="Bool (strict)"("Disabled"=w728) -> ()  [unwired: 2 in, 2 out]
            n790 = property on="SetOutputOffB" class="Bool (strict)"("Disabled"=w728) -> ()  [unwired: 2 in, 2 out]
            n791 = property on="SetVoltageAll" class="Bool (strict)"("Disabled"=w728) -> ()  [unwired: 2 in, 2 out]
            n792 = property on="SetCurrentAll" class="Bool (strict)"("Disabled"=w728) -> ()  [unwired: 2 in, 2 out]
            n793 = property on="DisconnectAll" class="Bool (strict)"("Disabled"=w728) -> ()  [unwired: 2 in, 2 out]
          }
        }
      }
    }
    n794 = call <vilib>:"General Error Handler.vi"("type of dialog (OK msg:1)"=u8 0 ("Disabled"), "error in (no error)"=w203) -> ()  [unwired: 14 out]
    n795 = Wait Until Next ms Multiple(millisecond multiple=u32 20) -> ()  [unwired: 1 out]
  }
  n796 = property on="Set Output ON All" class="Bool (strict)"("Disabled"=w24) -> (error out=w18:errorcluster)  [unwired: 2 in, 1 out]
  n797 = property on="SetCurrentAll" class="Bool (strict)"("Disabled"=w24) -> ()  [unwired: 2 in, 2 out]
  n798 = property on="AddChannel" class="Bool (strict)"("Disabled"=w24) -> ()  [unwired: 2 in, 2 out]
  n799 = property on="AddChannel" class="Bool (strict)"("Disabled"=u8 0) -> ()  [unwired: 2 in, 2 out]
  n800 = local write "текущий ист."(u8 0 ("текущий ист.")) -> ()
  n801 = local write "WriteToFile"(w26) -> ()
  n802 = local write "DisconnectChannel"(w26) -> ()
  n803 = local write "ConnectChannel"(w26) -> ()
  n804 = local write "SetCurrentB"(w26) -> ()
  n805 = local write "ReadFromFile"(w26) -> ()
  n806 = local write "AddChannel"(w26) -> ()
  n807 = local write "Quit"(w26) -> ()
  n808 = local write "SetCurrentAll"(w26) -> ()
  n809 = local write "SetVoltageAll"(w26) -> ()
  n810 = local write "DeleteChannel"(w26) -> ()
  n811 = local write "SetVoltageB"(w26) -> ()
  n812 = local write "SetOutputOnB"(w8) -> ()
  n813 = local write "ConnectAll"(w8) -> ()
  n814 = local write "SetOutputOffB"(w8) -> ()
  n815 = local write "DisconnectAll"(w8) -> ()
  n816 = property on="SelectedBuvSetVolB" class="Bool"("DisabledEnum"=T2."Enabled" ("Disabled")) -> ()  [unwired: 2 in, 2 out]
  n817 = disable-structure shown="Disabled" {
    frame Disabled {
      n818 = call <vilib>:"Application Directory.vi"() -> ("Application Directory"=w747:path)
      n819 = Build Path(base path=w747, name or relative path="BuvConfig.dat") -> (appended path=w744:path)
      n820 = Open/Create/Replace File(file path (use dialog)=w744, operation (0:open)=T3."open") -> (refnum out=w742:refnum<file>, error out=w743:errorcluster)  [unwired: 4 in, 1 out]
      n821 = Read from Text File(file (use dialog)=w742, error in=w743) -> (text=w739:string, error out=w734:errorcluster)  [unwired: 2 in, 2 out]
      n822 = Match Pattern(string=w739, regular expression="Z" ("string")) -> (before substring=w738:string, after substring=w735:string)  [unwired: 1 in, 2 out]
      n823 = Scan From String(input string=w735, error in=w734) -> (error out=w731:errorcluster, output 1=w736:dbl)  [unwired: 3 in, 2 out]
      n824 = local write "SelectedBuvOutVolt"(w736) -> ()
      n825 = Scan From String(input string=w738, error in=w731, default 1=u16 0 ("default value 1")) -> (error out=w733:errorcluster, output 1=w741:u16)  [unwired: 2 in, 2 out]
      n826 = local write item#-1(w741) -> ()
      n827 = case shown="No Error" w733 {
        selector: w733 -> [w791 w793]
        tunnel: [TRUE ("LoadPhase") FALSE ("LoadPhase")] -> w732
        tunnel: [w791 w793] -> w730
        frame No Error {
        }
        frame Error {
        }
      }
      "LoadPhase" <- w732
      n828 = while {
        tunnel: w730 -> [w748]
        stop <- FALSE stop-if-true
        n829 = flat-sequence {
          tunnel: [w761] -> w756
          tunnel: [w760] -> w755
          tunnel: w748 -> [w759]
          tunnel: w756 -> [w768]
          tunnel: w755 -> [w767]
          tunnel: [w766] -> w754
          tunnel: [w765] -> w753
          tunnel: w754 -> [w779]
          tunnel: [w778] -> w752
          tunnel: w753 -> [w777]
          tunnel: [w776] -> w751
          tunnel: w752 -> [w782]
          tunnel: w751 -> [w781]
          tunnel: [_] -> w750
          tunnel: [_] -> w749
          tunnel: w750 -> [w789]
          tunnel: w749 -> [w786]
          frame #0 {
            n830 = TCP Open Connection(address="172.16.21.81", remote port or service name=u16 4001, timeout ms (60000)=1000, error in (no error)=w759) -> (connection ID=w760:refnum<k5>, error out=w761:errorcluster)  [unwired: 1 in]
            "Buv con ID" <- w760
          }
          frame #1 {
            n831 = case shown="No Error" w768 {
              selector: w768 -> [w769 w775]
              tunnel: w767 -> [w770 w774]
              tunnel: [_ w775] -> w766
              tunnel: [_ w774] -> w765
              frame No Error {
                n832 = local read item#-1() -> (w772)
                n833 = Or(y=w772) -> (x .or. y?=w771:bool)  [unwired: 1 in]
                n834 = case shown="True" w771 {
                  tunnel: w770 -> [_ _]
                  tunnel: w769 -> [_ _]
                  frame False {
                  }
                  frame True {
                    # "Установка опорного напряжения"
                    n835 = local write item#-1(FALSE ("LoadPhase")) -> ()
                  }
                }
              }
              frame Error {
              }
            }
          }
          frame #2 {
          }
          frame #3 {
            n836 = case shown="Error" w782 {
              selector: w782 -> [_ w784]
              tunnel: w781 -> [_ w783]
              tunnel: [_ "*"] -> _
              tunnel: [_ w784] -> w780
              tunnel: [_ w783] -> _
              frame No Error {
              }
              frame Error {
              }
            }
          }
          frame #4 {
            n837 = case shown="Error" w786 {
              frame No Error {
              }
              frame Error {
                w790 = TRUE ("LoadPhase")
                n838 = local write "LoadPhase"(w790) -> ()
                n839 = local write item#-1(w790) -> ()
              }
            }
            n840 = TCP Close Connection(connection ID=w789) -> (error out=w788:errorcluster)  [unwired: 2 in, 1 out]
            n841 = call <vilib>:"General Error Handler.vi"("type of dialog (OK msg:1)"=0 ("milliseconds to wait"), "error in (no error)"=w788) -> ()  [unwired: 9 in, 5 out]
          }
        }
        n842 = Wait Until Next ms Multiple(millisecond multiple=u32 70) -> ()  [unwired: 1 out]
      }
    }
    frame Enabled {
    }
  }
  n843 = property on="DisconnectAll" class="Bool (strict)"(error in=w18, "Disabled"=w24) -> (error out=w17:errorcluster)  [unwired: 1 in, 1 out]
  n844 = property on="DisconnectChannel" class="Bool (strict)"("Disabled"=w24) -> (error out=w23:errorcluster)  [unwired: 2 in, 1 out]
  n845 = property on="WriteToFile" class="Bool (strict)"(error in=w17, "Disabled"=w24) -> (error out=w16:errorcluster)  [unwired: 1 in, 1 out]
  n846 = property on="SetCurrentB" class="Bool (strict)"(error in=w16, "Disabled"=w24) -> (error out=w15:errorcluster)  [unwired: 1 in, 1 out]
  n847 = property on="ConnectAll" class="Bool (strict)"(error in=w23, "Disabled"=w24) -> (error out=w22:errorcluster)  [unwired: 1 in, 1 out]
  n848 = property on="Quit" class="Bool (strict)"(error in=w15, "Disabled"=w24) -> (error out=w14:errorcluster)  [unwired: 1 in, 1 out]
  n849 = property on="ReadFromFile" class="Bool (strict)"(error in=w22, "Disabled"=w24) -> (error out=w21:errorcluster)  [unwired: 1 in, 1 out]
  n850 = property on="SetOutputOnB" class="Bool (strict)"(error in=w14, "Disabled"=w24) -> (error out=w13:errorcluster)  [unwired: 1 in, 1 out]
  n851 = property on="ConnectChannel" class="Bool (strict)"(error in=w21, "Disabled"=w24) -> (error out=w20:errorcluster)  [unwired: 1 in, 1 out]
  n852 = property on="SetVoltageB" class="Bool (strict)"(error in=w13, "Disabled"=w24) -> (error out=w12:errorcluster)  [unwired: 1 in, 1 out]
  n853 = property on="SetOutputOffB" class="Bool (strict)"(error in=w12, "Disabled"=w24) -> ()  [unwired: 1 in, 2 out]
  n854 = property on="DeleteChannel" class="Bool (strict)"(error in=w20, "Disabled"=w24) -> (error out=w19:errorcluster)  [unwired: 1 in, 1 out]
  n855 = property on="SetVoltageAll" class="Bool (strict)"(error in=w19, "Disabled"=w24) -> ()  [unwired: 1 in, 2 out]
  n856 = event shown="[0] \"Quit\": Value Change" {
    selector: _ -> [_]
    dyn-events: _ -> [_]
    timeout: _ -> [_]
    event "Quit": Value Change {
      n857 = event-data() -> ()  [unwired: 1 in, 1 out]
      n858 = flat-sequence {
        frame #0 {
          w800 = T4 0 items=["no dialog", "OK message", "continue or stop message", "OK message + warnings", "continue/stop + warnings"] ("type of dialog (OK msg:1)")
          n859 = local read "BuvCtrlVI_VIRef"() -> (w797:refnum<vi>[])
          n860 = Array Size(array=w797) -> (size(s)=w799:i32)
          n861 = for {
            N: w799 -> [_]
            tunnel: [w821] -> w798 mode=indexing
            tunnel: w797 -> [w820]
            i -> [w822]
            n862 = Index Array(array=w820, index=w822) -> (element=w814:refnum<vi>)
            n863 = To Variant(anything=TRUE ("ConnectChannel")) -> (Variant=w817:variant)
            n864 = invoke on="Invoke Node" class="VI" method="Ctrl Val.Set"(reference=w814, "Control Name"="TCP disconnect", "Value"=w817) -> (reference out=w816:refnum<vi>, error out=w815:errorcluster)  [unwired: 2 in, 3 out]
            n865 = flat-sequence {
              tunnel: [w825] -> w813
              tunnel: w816 -> [w825]
              tunnel: [w824] -> w812
              tunnel: w815 -> [w824]
              frame #0 {
                n866 = Wait (ms)(milliseconds to wait=u32 100) -> ()  [unwired: 1 out]
              }
            }
            n867 = invoke class="VI" method="Abort VI"(reference=w813, error in=w812) -> (error out=w821:errorcluster)  [unwired: 1 in, 2 out]
          }
          n868 = local read "TctrlConID"() -> (w796:refnum<k5>)
          n869 = disable-structure shown="Disabled" {
            disable-tunnel: [w804 _] -> w802
            frame Disabled {
              n870 = local read "Measure_VI"() -> (w803:refnum<vi>[])
              n871 = Array Size(array=w803) -> (size(s)=w805:i32)
              n872 = for {
                N: w805 -> [_]
                tunnel: [w807] -> w804 mode=indexing
                tunnel: w803 -> [w806]
                i -> [w808]
                n873 = Index Array(array=w806, index=w808) -> (element=w810:refnum<vi>)
                n874 = invoke class="VI" method="Ctrl Val.Set"(reference=w810, "Control Name"="Connect", "Value"=FALSE ("OK Button")) -> (error out=w807:errorcluster)  [unwired: 2 in, 4 out]
              }
            }
            frame Enabled {
            }
          }
          n875 = TCP Close Connection(connection ID=w796) -> (error out=w795:errorcluster)  [unwired: 2 in, 1 out]
          n876 = Merge Errors(w802, w798, w795) -> (w801:errorcluster)
          n877 = call <vilib>:"General Error Handler.vi"("type of dialog (OK msg:1)"=w800, "error in (no error)"=w801) -> ()  [unwired: 9 in, 5 out]
        }
        frame #1 {
          n878 = Wait (ms)(milliseconds to wait=u32 100) -> ()  [unwired: 1 out]
        }
        frame #2 {
          n879 = Stop(stop? (T)=TRUE) -> ()
        }
      }
    }
  }
  n880 = while {
    stop <- FALSE stop-if-true
    w831 = T4 0 items=["no dialog", "OK message", "continue or stop message", "OK message + warnings", "continue/stop + warnings"] ("type of dialog (OK msg:1)")
    # "БУВы"
    n881 = event shown="[2] \"AddNewBuv\": Value Change" {
      selector: _ -> [_ _ _ _ _ _ _]
      dyn-events: _ -> [_ _ _ _ _ _ _]
      timeout: _ -> [_ _ _ _ _ _ _]
      tunnel: [w834 w847 w864 w890 w911 w948 w1013] -> w830
      event "SelectedBuvSetVolB": Value Change {
        n882 = event-data() -> ()  [unwired: 1 in, 1 out]
        n883 = property on="Buv Table" class="MCListbox (strict)"() -> ("Value"=w841:i32)  [unwired: 2 in, 2 out]
        n884 = local read "BuvCtrlVI_VIRef"() -> (w836:refnum<vi>[])
        n885 = Index Array(array=w836, index=w841) -> (element=w837:refnum<vi>)
        n886 = To Variant(anything="SelectedBuvOutVolt") -> (Variant=w842:variant)
        n887 = invoke class="VI" method="Ctrl Val.Set"(reference=w837, "Control Name"="SetVoltage", "Value"=w842) -> (reference out=w839:refnum<vi>, error out=w840:errorcluster)  [unwired: 2 in, 3 out]
        n888 = To Variant(anything=TRUE ("ConnectChannel")) -> (Variant=w843:variant)
        n889 = invoke class="VI" method="Ctrl Val.Set"(reference=w839, error in=w840, "Control Name"="SetV", "Value"=w843) -> (error out=w834:errorcluster)  [unwired: 1 in, 4 out]
      }
      event "SelectedBuvOutStateB": Value Change {
        # "ВКЛ/ВЫКЛ силовую часть выбранного БУВа"
        n890 = event-data() -> ("NewVal"=w845:bool)  [unwired: 1 in]
        n891 = property on="Buv Table" class="MCListbox (strict)"() -> ("Value"=w850:i32)  [unwired: 2 in, 2 out]
        n892 = local read "BuvCtrlVI_VIRef"() -> (w848:refnum<vi>[])
        n893 = Index Array(array=w848, index=w850) -> (element=w846:refnum<vi>)
        n894 = case shown="True" w845 {
          tunnel: [w853 w856] -> w851
          tunnel: ["SetOutON" ("Control Name") "SetOutOFF" ("Control Name")] -> w849
          frame True {
            n895 = To Variant(anything=TRUE ("ConnectChannel")) -> (Variant=w853:variant)
          }
          frame False {
            n896 = To Variant(anything=TRUE ("ConnectChannel")) -> (Variant=w856:variant)
          }
        }
        n897 = invoke class="VI" method="Ctrl Val.Set"(reference=w846, "Control Name"=w849, "Value"=w851) -> (error out=w847:errorcluster)  [unwired: 2 in, 4 out]
      }
      event "AddNewBuv": Value Change {
        n898 = event-data() -> ("OldVal"=w870:bool)  [unwired: 1 in]
        n899 = local write "AddNewBuv"(w870) -> ()
        n900 = local read "BuvCtrlVI_VIRef"() -> (w869:refnum<vi>[])
        n901 = local read "BuvNameArr"() -> (w867:string[])
        n902 = local read "Buv IP"() -> (w863:string[])
        n903 = call "AddNewBuv.vi"("Num of Buvs in"="Num of Buvs", "New BuV IP"="NewBuvIP", "Voltage"="0", "Name Arr IN"=w867, "New BuV name"="NewBuvName", "Buv IP arr"=w863, "BuvCtrlVI_VIRef"=w869) -> ("BuvCtrlVI_VIRefOut"=w868:refnum<vi>[], "Num of Buvs out"=w858:u8, "Name Out"=w865:string[], "Buv Ip Out"=w866:string[], "error out"=w864:errorcluster)  [unwired: 16 in]
        n904 = local write "BuvNameArr"(w865) -> ()
        n905 = local write "BuvCtrlVI_VIRef"(w868) -> ()
        n906 = local write "Num of Buvs"(w858) -> ()
        n907 = local write "Buv IP"(w866) -> ()
      }
      event "DeleteBuv": Value Change {
        n908 = event-data() -> ("OldVal"=w894:bool)  [unwired: 1 in]
        n909 = property on="Buv Table" class="MCListbox (strict)"() -> ("Value"=w871:i32)  [unwired: 2 in, 2 out]
        n910 = local read "Num of Buvs"() -> (w892:u8)
        n911 = local write "DeleteBuv"(w894) -> ()
        n912 = local read "BuvCtrlVI_VIRef"() -> (w893:refnum<vi>[])
        n913 = Bundle "Connet status"("Value"=w871, "milliseconds to wait"=5) -> (w872:cluster{"Value":i32, "milliseconds to wait":i32})  [unwired: 1 in]
        n914 = Decrement(x=w892) -> (x-1=w891:u8)
        n915 = property on="Buv Table" class="MCListbox (strict)"("ActiveCell"=w872, "CellBG"=u32 16777226) -> ()  [unwired: 2 in, 2 out]
        n916 = Index Array(array=w893, index=w871) -> (element=w887:refnum<vi>)
        n917 = To Variant(anything=TRUE ("ConnectChannel")) -> (Variant=w885:variant)
        n918 = local write "Num of Buvs"(w891) -> ()
        n919 = invoke on="Invoke Node" class="VI" method="Ctrl Val.Set"(reference=w887, "Control Name"="TCP disconnect", "Value"=w885) -> (reference out=w883:refnum<vi>, error out=w881:errorcluster)  [unwired: 2 in, 3 out]
        n920 = Bundle "Out status"("Value"=w871, "milliseconds to wait"=4) -> (w875:cluster{"Value":i32, "milliseconds to wait":i32})  [unwired: 1 in]
        n921 = flat-sequence {
          tunnel: [w897] -> w884
          tunnel: w883 -> [w897]
          tunnel: [w896] -> w882
          tunnel: w881 -> [w896]
          frame #0 {
            n922 = Wait (ms)(milliseconds to wait=u32 100) -> ()  [unwired: 1 out]
          }
        }
        n923 = property on="Buv Table" class="MCListbox (strict)"("ActiveCell"=w875, "CellBG"=u32 16777226) -> ()  [unwired: 2 in, 2 out]
        n924 = invoke class="VI" method="Abort VI"(reference=w884, error in=w882) -> (error out=w890:errorcluster)  [unwired: 1 in, 2 out]
        n925 = Equal To 0?(x=w871) -> (x = 0?=w889:bool)
        n926 = Bundle "Fault status"("Value"=w871, "milliseconds to wait"=6) -> (w876:cluster{"Value":i32, "milliseconds to wait":i32})  [unwired: 1 in]
        n927 = case shown="False" w889 {
          tunnel: w871 -> [w905 _]
          frame False {
            n928 = local read "BuvCtrlVI_VIRef"() -> (w903:refnum<vi>[])
            n929 = local read "BuvNameArr"() -> (w902:string[])
            n930 = local read "Buv IP"() -> (w901:string[])
            n931 = Delete From Array(array=w903, length=1, index=w905) -> (array with subset deleted=w900:refnum<vi>[])  [unwired: 1 out]
            n932 = Delete From Array(array=w902, length=1, index=w905) -> (array with subset deleted=w899:string[])  [unwired: 1 out]
            n933 = Delete From Array(array=w901, length=1, index=w905) -> (array with subset deleted=w898:string[])  [unwired: 1 out]
            n934 = local write "BuvCtrlVI_VIRef"(w900) -> ()
            n935 = local write "BuvNameArr"(w899) -> ()
            n936 = local write "Buv IP"(w898) -> ()
          }
          frame True {
            w908 = string[] [] ("BuvNameArr")
            n937 = local write "BuvCtrlVI_VIRef"(refnum<vi>[] [] ("BuvCtrlVI_VIRef")) -> ()
            n938 = local write "BuvNameArr"(w908) -> ()
            n939 = local write "Buv IP"(w908) -> ()
          }
        }
        n940 = property on="Buv Table" class="MCListbox (strict)"("ActiveCell"=w876, "CellBG"=u32 16777226) -> ()  [unwired: 2 in, 2 out]
      }
      event "Buv Table": Mouse Down {
        # "Работа с выбранным источником БУВ"
        n941 = event-data() -> ()  [unwired: 1 in, 1 out]
        n942 = property on="Buv Table" class="MCListbox (strict)"() -> ("ItemNames"=w912:string[][])  [unwired: 2 in, 2 out]
        n943 = property on="Buv Table" class="MCListbox (strict)"() -> ("Value"=w910:i32)  [unwired: 2 in, 2 out]
        n944 = Index Array(array=w912, index (row)=w910) -> (element=w913:string[])  [unwired: 1 in]
        n945 = Empty Array?(array=w913) -> (empty?=w914:bool)
        n946 = case shown="False" w914 {
          tunnel: w913 -> [w918 _]
          tunnel: [w916 _] -> w911
          tunnel: w910 -> [w915 _]
          frame False {
            n947 = flat-sequence {
              tunnel: w918 -> [w929]
              tunnel: [w929] -> w919
              tunnel: [w927] -> w917
              tunnel: w915 -> [w923]
              tunnel: w919 -> [w939]
              tunnel: w917 -> [w934]
              tunnel: [w933] -> w916
              frame #0 {
                n948 = Bundle "Out status"("Value"=w923, "index"=4) -> (w921:cluster{"Value":i32, "index":i32})  [unwired: 1 in]
                n949 = Index Array(array=w929, index=0) -> (element=w930:string)
                n950 = property on="Buv Table" class="MCListbox (strict)"("ActiveCell"=w921) -> (error out=w926:errorcluster)  [unwired: 2 in, 1 out]
                n951 = Scan From String(format string="%f", input string=w930) -> (error out=w927:errorcluster, output 1=→"текущий ист. БУВ":u8)  [unwired: 3 in, 2 out]
                n952 = property on="Buv Table" class="MCListbox (strict)"(error in=w926) -> ("CellBG"=w924:u32)  [unwired: 1 in, 2 out]
                n953 = Equal?(x=u32 5895331, y=w924) -> (x = y?=w920:bool)
                n954 = property on="SelectedBuvOutStateB" class="Bool (strict)"("Value"=w920) -> ()  [unwired: 2 in, 2 out]
              }
              frame #1 {
                n955 = Index Array(array=w939, index=2) -> (element=w937:string)
                n956 = Scan From String(format string="%f", input string=w937, error in=w934) -> (error out=w933:errorcluster, output 1=w935:dbl)  [unwired: 2 in, 2 out]
                n957 = local write "SelectedBuvOutVolt"(w935) -> ()
              }
            }
          }
          frame True {
          }
        }
      }
      event "ReadFromFile Buv": Value Change {
        n958 = event-data() -> ("OldVal"=w947:bool)  [unwired: 1 in]
        n959 = call "File Dialog2"("start path"=path "C:/", "prompt"="Укажите конфигурационный файл" ("prompt (Open existing file)"), "pattern (all files)"="*.dat", "pattern label"="Настройки ЛЖФ") -> ("selected path"=w945:path, "error out"=w942:errorcluster)  [unwired: 8 in, 2 out]
        n960 = Read from Text File(file (use dialog)=w945, count=-1, error in=w942) -> (text=w953:string[], cancelled=w949:bool, error out=w954:errorcluster)  [unwired: 2 out]
        n961 = Not(x=w949) -> (.not. x?=w951:bool)
        n962 = Not(x=w954) -> (.not. x?=w952:bool)
        n963 = And(x=w951, y=w952) -> (x .and. y?=w950:bool)
        n964 = local write "ReadFromFile Buv"(w947) -> ()
        n965 = case shown="True" w950 {
          tunnel: w953 -> [_ w962]
          tunnel: [w956 w960] -> w955
          tunnel: w954 -> [w957 w958]
          frame False {
            n966 = Build Array(w957) -> (w956:errorcluster[])
          }
          frame True {
            n967 = flat-sequence {
              tunnel: w962 -> [w965]
              tunnel: [w965] -> w961
              tunnel: [w964] -> w959
              tunnel: w958 -> [w964]
              tunnel: w961 -> [w970]
              tunnel: [w969] -> w960
              tunnel: w959 -> [w968]
              frame #0 {
                w966 = string[] [] ("Buv IP")
                n968 = local write "Num of Buvs"(u8 0 ("Num of Buvs")) -> ()
                "Buv IP" <- w966
                "BuvNameArr" <- w966
                "BuvCtrlVI_VIRef" <- refnum<vi>[] [] ("BuvCtrlVI_VIRef")
              }
              frame #1 {
                n969 = Index Array(array=w970, index=0) -> (element=w972:string)
                n970 = Decimal String To Number(string=w972) -> (number=w971:i32)  [unwired: 3 out]
                n971 = for {
                  N: w971 -> [_]
                  tunnel: w970 -> [w997]
                  tunnel: [w989] -> w969 mode=indexing
                  tunnel: w968 -> [w990]
                  i -> [w996]
                  # "Добавление нового БУВа"
                  n972 = Increment(x=w996) -> (x+1=w974:i32)
                  n973 = Index Array(array=w997, index=w974) -> (element=w979:string)
                  n974 = Spreadsheet String To Array(format string="%s", spreadsheet string=w979, array type (2D Dbl)=string[] [] ("GlobalInAdress")) -> (array=w985:string[])  [unwired: 1 out]
                  n975 = local read "BuvCtrlVI_VIRef"() -> (w995:refnum<vi>[])
                  n976 = local read "Buv IP"() -> (w988:string[])
                  n977 = local read "BuvNameArr"() -> (w987:string[])
                  n978 = local read "Num of Buvs"() -> (w986:u8)
                  n979 = Index Array "Name"(array=w985, index=0) -> (element=w975:string)
                  n980 = Index Array "IP"(array=w985, index=1) -> (element=w978:string)
                  n981 = Index Array "SetV"(array=w985, index=2) -> (element=w977:string)
                  n982 = call "AddNewBuv.vi"("Num of Buvs in"=w986, "New BuV IP"=w978, "Voltage"=w977, "error in"=w990, "Name Arr IN"=w987, "New BuV name"=w975, "Buv IP arr"=w988, "BuvCtrlVI_VIRef"=w995) -> ("BuvCtrlVI_VIRefOut"=w994:refnum<vi>[], "Num of Buvs out"=w976:u8, "Name Out"=w992:string[], "Buv Ip Out"=w993:string[], "error out"=w991:errorcluster)  [unwired: 15 in]
                  n983 = local write "BuvCtrlVI_VIRef"(w994) -> ()
                  n984 = flat-sequence {
                    tunnel: [w998] -> w989
                    tunnel: w991 -> [w998]
                    frame #0 {
                      n985 = Wait (ms)(milliseconds to wait=u32 50) -> ()  [unwired: 1 out]
                    }
                  }
                  n986 = local write "BuvNameArr"(w992) -> ()
                  n987 = local write "Buv IP"(w993) -> ()
                  n988 = local write "Num of Buvs"(w976) -> ()
                }
              }
            }
          }
        }
        n989 = Merge Errors(w955) -> (w948:errorcluster)
      }
      event "WriteToFile Buv": Value Change {
        w1000 = "Настройки ЛЖФ " ("default name")
        # "Запись конфигурации БУВов в файл"
        n990 = event-data() -> ("OldVal"=w1018:bool)  [unwired: 1 in]
        n991 = local read "BuvCtrlVI_VIRef"() -> (w1017:refnum<vi>[])
        n992 = local write "WriteToFile Buv"(w1018) -> ()
        n993 = Array Size(array=w1017) -> (size(s)=w1016:i32)
        n994 = Number To Decimal String(number=w1016) -> (decimal integer string=w1008:string)  [unwired: 1 out]
        n995 = for {
          N: w1016 -> [_]
          tunnel: [w1021] -> w1015 mode=indexing
          tunnel: [w1019] -> w1006 mode=indexing
          i -> [w1025]
          w1023 = "\t"
          n996 = local read "BuvCtrlVI_VIRef"() -> (w1029:refnum<vi>[])
          n997 = Index Array(array=w1029, index=w1025) -> (element=w1028:refnum<vi>)
          n998 = invoke class="VI" method="Ctrl Val.Get"(reference=w1028, "Control Name"="SetVstr") -> (error out=w1031:errorcluster, "Get Control Value Variant"=w1030:variant)  [unwired: 2 in, 2 out]
          n999 = local read "BuvNameArr"() -> (w1033:string[])
          n1000 = local read "Buv IP"() -> (w1032:string[])
          n1001 = Index Array(array=w1033, index=w1025) -> (element=w1034:string)
          n1002 = Index Array(array=w1032, index=w1025) -> (element=w1024:string)
          n1003 = Variant To Data(error in=w1031, type="" ("Control Name"), Variant=w1030) -> (data=w1022:string, error out=w1021:errorcluster)
          n1004 = Concatenate Strings(w1034, w1023, w1024, w1023, w1022, "\r\n") -> (w1019:string)
        }
        n1005 = Merge Errors(w1015) -> (w1014:errorcluster)
        n1006 = call "File Dialog"("start path"=path "C:/", "prompt"="Укажите имя и директорию файла" ("prompt (Choose or enter file path)"), "default name"=w1000, "pattern (all files)"="*.dat", "pattern label"=w1000) -> ("selected path"=w1005:path, "error out"=w1004:errorcluster)  [unwired: 7 in, 2 out]
        n1007 = Concatenate Strings(w1008, "\r\n", w1006) -> (w1007:string)
        n1008 = Write to Text File(file (use dialog)=w1005, text=w1007, error in=w1004) -> (refnum out=w1011:refnum<file>, error out=w1012:errorcluster)  [unwired: 2 out]
        n1009 = Close File(refnum=w1011, error in=w1012) -> (error out=w1010:errorcluster)  [unwired: 1 out]
        n1010 = Merge Errors(w1010, w1014) -> (w1013:errorcluster)
      }
    }
    n1011 = call <vilib>:"General Error Handler.vi"("type of dialog (OK msg:1)"=w831, "error in (no error)"=w830) -> ("message"=→"message event":string)  [unwired: 9 in, 4 out]
    n1012 = Wait Until Next ms Multiple(millisecond multiple=u32 20) -> ()  [unwired: 1 out]
  }
  n1013 = while {
    stop <- FALSE stop-if-true
    # "БУВы. Обновление данных и вывод в таблицу"
    n1014 = local read "BuvCtrlVI_VIRef"() -> (w1039:refnum<vi>[])
    n1015 = Wait Until Next ms Multiple(millisecond multiple=u32 20) -> ()  [unwired: 1 out]
    n1016 = Array Size(array=w1039) -> (size(s)=w1035:i32)
    n1017 = disable-structure shown="Enabled" {
      disable-tunnel: [w1041 TRUE] -> w1036
      disable-tunnel: w1035 -> [w1040 _]
      frame Disabled {
        n1018 = Not Equal To 0?(x=w1040) -> (x != 0?=w1041:bool)
      }
      frame Enabled {
      }
    }
    n1019 = case shown="True" w1036 {
      tunnel: w1035 -> [_ w1067]
      tunnel: w1039 -> [_ w1066]
      frame False {
      }
      frame True {
        w1054 = T4 0 items=["no dialog", "OK message", "continue or stop message", "OK message + warnings", "continue/stop + warnings"] ("type of dialog (OK msg:1)")
        w1047 = string[] [] ("GlobalInAdress")
        n1020 = for {
          N: w1067 -> [_]
          tunnel: w1066 -> [w1162]
          shift-right: [w1140] -> w1064
          shift-left: w1047 -> [w1142]
          shift-right: [w1138] -> w1062
          shift-left: w1047 -> [w1137]
          shift-right: [w1133] -> w1049
          shift-left: w1047 -> [w1132]
          shift-right: [w1131] -> w1048
          shift-left: w1047 -> [w1130]
          shift-right: [w1129] -> w1050
          shift-left: w1047 -> [w1128]
          shift-right: [w1127] -> w1063
          shift-left: w1047 -> [w1126]
          tunnel: [w1118] -> w1060 mode=indexing
          tunnel: [w1117] -> w1058 mode=indexing
          tunnel: [w1116] -> w1056 mode=indexing
          tunnel: [w1110] -> w1059 mode=indexing
          tunnel: [w1115] -> w1057 mode=indexing
          shift-right: [w1103] -> w1046
          shift-left: w1047 -> [w1102]
          tunnel: [w1101] -> w1045 mode=indexing
          i -> [w1164]
          n1021 = Index Array(array=w1162, index=w1164) -> (element=w1105:refnum<vi>)
          n1022 = invoke class="VI" method="Ctrl Val.Get"(reference=w1105, "Control Name"="ReadV") -> (error out=w1147:errorcluster, "Get Control Value Variant"=w1157:variant)  [unwired: 2 in, 2 out]
          n1023 = invoke class="VI" method="Ctrl Val.Get"(reference=w1105, "Control Name"="ReadI") -> (error out=w1146:errorcluster, "Get Control Value Variant"=w1159:variant)  [unwired: 2 in, 2 out]
          n1024 = invoke class="VI" method="Ctrl Val.Get"(reference=w1105, "Control Name"="SetVoltage") -> (error out=w1143:errorcluster, "Get Control Value Variant"=w1149:variant)  [unwired: 2 in, 2 out]
          n1025 = invoke class="VI" method="Ctrl Val.Get"(reference=w1105, "Control Name"="Active_num") -> (error out=w1144:errorcluster, "Get Control Value Variant"=w1152:variant)  [unwired: 2 in, 2 out]
          n1026 = invoke class="VI" method="Ctrl Val.Get"(reference=w1105, "Control Name"="status cluster") -> (error out=w1145:errorcluster, "Get Control Value Variant"=w1155:variant)  [unwired: 2 in, 2 out]
          n1027 = invoke class="VI" method="Ctrl Val.Get"(reference=w1105, "Control Name"="ErrMessage") -> (error out=w1109:errorcluster, "Get Control Value Variant"=w1108:variant)  [unwired: 2 in, 2 out]
          n1028 = Variant To Data(error in=w1147, type="" ("Control Name"), Variant=w1157) -> (data=w1141:string, error out=w1118:errorcluster)
          n1029 = Variant To Data(error in=w1146, type="" ("Control Name"), Variant=w1159) -> (data=w1139:string, error out=w1117:errorcluster)
          n1030 = Variant To Data(error in=w1143, type=0.0 ("Active_num"), Variant=w1149) -> (data=w1113:dbl, error out=w1111:errorcluster)
          n1031 = Variant To Data(error in=w1145, type=cluster{bool, bool, bool} {FALSE, FALSE, FALSE} ("status cluster"), Variant=w1155) -> (data=w1134:cluster{bool, bool, bool}, error out=w1116:errorcluster)
          n1032 = Variant To Data(error in=w1144, type=i16 0 ("Active_num"), Variant=w1152) -> (data=w1124:i16, error out=w1115:errorcluster)
          n1033 = Variant To Data(error in=w1109, type="" ("Control Name"), Variant=w1108) -> (data=w1104:string, error out=w1101:errorcluster)
          n1034 = Unbundle(w1134) -> (w1136:bool, w1135:bool)  [unwired: 1 out]
          n1035 = Number To Decimal String(number=w1124, width (-)=i16 1) -> (decimal integer string=w1123:string)
          n1036 = Boolean To (0,1)(Boolean=w1136) -> (0, 1=w1099:i16)
          n1037 = Boolean To (0,1)(Boolean=w1135) -> (0, 1=w1122:i16)
          n1038 = Format Into String(format string="%.1f", error in=w1111, w1113) -> (resulting string=w1112:string, error out=w1110:errorcluster)  [unwired: 1 in]
          n1039 = Number To Decimal String(number=w1099, width (-)=i16 1) -> (decimal integer string=w1119:string)
          n1040 = Number To Decimal String(number=w1122, width (-)=i16 1) -> (decimal integer string=w1120:string)
          n1041 = Build Array (concatenate) "Buvs current"(w1137, w1139) -> (w1138:string[])
          n1042 = Build Array (concatenate) "Err"(w1102, w1104) -> (w1103:string[])
          n1043 = Build Array (concatenate) "Buvs con status"(w1128, w1123) -> (w1129:string[])
          n1044 = Build Array (concatenate) "Buvs set V"(w1126, w1112) -> (w1127:string[])
          n1045 = Build Array (concatenate) "Buvs read voltage"(w1142, w1141) -> (w1140:string[])
          n1046 = Build Array (concatenate) "Buvs fault"(w1130, w1120) -> (w1131:string[])
          n1047 = Build Array (concatenate) "Buvs out state"(w1132, w1119) -> (w1133:string[])
        }
        "Error BuvVIctrl" <- w1046
        n1048 = local read "BuvNameArr"() -> (w1044:string[])
        n1049 = disable-structure shown="Enabled" {
          disable-tunnel: w1044 -> [w1069 w1070]
          disable-tunnel: [w1068 w1070] -> w1043
          frame Disabled {
            n1050 = Reverse 1D Array(array=w1069) -> (reversed array=w1068:string[])
          }
          frame Enabled {
          }
        }
        n1051 = Merge Errors(w1060, w1059, w1058, w1057, w1056, w1045) -> (w1055:errorcluster)
        n1052 = Build Array(w1043, w1064, w1063, w1062) -> (w1065:string[][])
        n1053 = call <vilib>:"General Error Handler.vi"("type of dialog (OK msg:1)"=w1054, "error in (no error)"=w1055) -> ("message"=→"message upd":string)  [unwired: 9 in, 4 out]
        n1054 = Transpose 2D Array(2D array=w1065) -> (transposed array=w1061:string[][])
        n1055 = property on="Buv Table" class="MCListbox (strict)"("ItemNames"=w1061) -> ()  [unwired: 2 in, 2 out]
        n1056 = local read "BuvCtrlVI_VIRef"() -> (w1052:refnum<vi>[])
        n1057 = Array Size(array=w1052) -> (size(s)=w1051:i32)
        n1058 = for {
          N: w1051 -> [_]
          tunnel: w1050 -> [w1096]
          tunnel: w1049 -> [w1081]
          tunnel: w1048 -> [w1072]
          i -> [w1071]
          n1059 = Index Array(array=w1096, index=w1071) -> (element=w1095:string)
          n1060 = Index Array(array=w1081, index=w1071) -> (element=w1084:string)
          n1061 = Index Array(array=w1072, index=w1071) -> (element=w1078:string)
          n1062 = Equal?(x="1", y=w1095) -> (x = y?=w1093:bool)
          n1063 = Equal?(x="1", y=w1084) -> (x = y?=w1086:bool)
          n1064 = Equal?(x="1", y=w1078) -> (x = y?=w1076:bool)
          n1065 = Select(t=u32 5895331, s=w1093, f=u32 15329769) -> (s? t:f=w1090:u32)
          n1066 = Select(t=u32 5895331, s=w1086, f=u32 15329769) -> (s? t:f=w1089:u32)
          n1067 = Select(t=u32 16711680, s=w1076, f=u32 16448250) -> (s? t:f=w1073:u32)
          n1068 = Bundle "Connet status"(w1071, "milliseconds to wait"=5) -> (w1098:cluster{i32, "milliseconds to wait":i32})  [unwired: 1 in]
          n1069 = Bundle "Out status"(w1071, "milliseconds to wait"=4) -> (w1082:cluster{i32, "milliseconds to wait":i32})  [unwired: 1 in]
          n1070 = Bundle "Fault status"(w1071, "milliseconds to wait"=6) -> (w1080:cluster{i32, "milliseconds to wait":i32})  [unwired: 1 in]
          n1071 = property on="Buv Table" class="MCListbox (strict)"("ActiveCell"=w1098, "CellBG"=w1090) -> ()  [unwired: 2 in, 2 out]
          n1072 = property on="Buv Table" class="MCListbox (strict)"("ActiveCell"=w1082, "CellBG"=w1089) -> ()  [unwired: 2 in, 2 out]
          n1073 = property on="Buv Table" class="MCListbox (strict)"("ActiveCell"=w1080, "CellBG"=w1073) -> ()  [unwired: 2 in, 2 out]
        }
      }
    }
  }
  n1074 = while {
    stop <- FALSE stop-if-true
    w1170 = T4 0 items=["no dialog", "OK message", "continue or stop message", "OK message + warnings", "continue/stop + warnings"] ("type of dialog (OK msg:1)")
    n1075 = TCP Open Connection(address="172.16.21.67", remote port or service name=u16 4001, timeout ms (60000)=1000) -> (connection ID=w1175:refnum<k5>, error out=w1174:errorcluster)  [unwired: 1 in, 1 out]
    "TctrlConID" <- w1175
    n1076 = while {
      tunnel: w1175 -> [w1192]
      tunnel: w1174 -> [w1191]
      tunnel: [w1181] -> w1168
      tunnel: [w1180] -> w1165
      stop <- w1180 stop-if-true
      n1077 = call "LU20_T_Control.vi"("connection ID in"=w1192, "error IN"=w1191) -> ("T cluster"=w1189:T5, "alarm cluster"=w1190:T6, "connection ID out"=w1182:refnum<k5>, "error OUT"=w1183:errorcluster)  [unwired: 14 in]
      n1078 = Unbundle By Name "Temperature"(w1189) -> ("T1"=→"К1":dbl, "T2"=→"К2":dbl, "T3"=→"K3":dbl, "T4"=→"Напор \nобщий":dbl, "T5"=→"Cлив \nобщий":dbl)
      n1079 = Unbundle By Name(w1190) -> ()  [unwired: 5 out]
      n1080 = case shown="Error" w1183 {
        selector: w1183 -> [_ w1203]
        tunnel: w1182 -> [w1195 w1206]
        tunnel: [w1193 w1204] -> w1181
        tunnel: [_ w1201] -> w1180
        frame No Error {
          n1081 = flat-sequence {
            tunnel: w1195 -> [w1196]
            tunnel: [w1196] -> w1194
            tunnel: w1194 -> [w1199]
            tunnel: [w1199] -> w1193
            frame #0 {
              n1082 = property on="T upd fl" class="Bool (strict)"() -> ("Value"=w1197:bool)  [unwired: 2 in, 2 out]
              n1083 = Not(x=w1197) -> (.not. x?=w1198:bool)
              n1084 = property on="T upd fl" class="Bool (strict)"("Value"=w1198) -> ()  [unwired: 2 in, 2 out]
            }
            frame #1 {
              n1085 = Wait (ms)(milliseconds to wait=u32 1000) -> ()  [unwired: 1 out]
            }
          }
        }
        frame Error {
          n1086 = flat-sequence {
            tunnel: w1206 -> [w1209]
            tunnel: [w1209] -> w1205
            tunnel: w1203 -> [w1208]
            tunnel: [w1207] -> w1202
            tunnel: w1205 -> [w1212]
            tunnel: [w1212] -> w1204
            tunnel: w1202 -> [w1211]
            tunnel: [w1211] -> w1201
            frame #0 {
              n1087 = property on="T upd fl" class="Bool (strict)"(error in=w1208, "Value"=FALSE ("T upd fl")) -> (error out=w1207:errorcluster)  [unwired: 1 in, 1 out]
            }
            frame #1 {
              n1088 = Wait (ms)(milliseconds to wait=u32 1000) -> ()  [unwired: 1 out]
            }
          }
        }
      }
    }
    n1089 = flat-sequence {
      tunnel: [w1178] -> w1167
      tunnel: w1168 -> [w1178]
      tunnel: [w1177] -> w1166
      tunnel: w1165 -> [w1177]
      frame #0 {
        n1090 = Wait (ms)(milliseconds to wait=u32 1000) -> ()  [unwired: 1 out]
      }
    }
    n1091 = TCP Close Connection(connection ID=w1167, error in (no error)=w1166) -> (error out=w1169:errorcluster)  [unwired: 1 in, 1 out]
    n1092 = call <vilib>:"General Error Handler.vi"("type of dialog (OK msg:1)"=w1170, "error in (no error)"=w1169) -> ()  [unwired: 9 in, 5 out]
  }
  n1093 = local write "BuvNameArr"(w7) -> ()
  n1094 = local write "Buv IP"(w7) -> ()
  n1095 = for {
    N: 20 -> [_]
    i -> [w1215]
    w1214 = T7 {"Font Name"="Application font", "Size"=27, "Bold"=TRUE, "Italic"=FALSE, "Underline"=FALSE, "Strikeout"=FALSE, "Color"=5011} ("Active Cell:Cell Font")
    # "Очистка таблицы при вкл, шрифты -БУВы"
    n1096 = Bundle "Connet status"(w1215, "milliseconds to wait"=5) -> (w1232:cluster{i32, "milliseconds to wait":i32})  [unwired: 1 in]
    n1097 = Bundle "Out status"(w1215, "milliseconds to wait"=4) -> (w1229:cluster{i32, "milliseconds to wait":i32})  [unwired: 1 in]
    n1098 = Bundle "Fault status"(w1215, "milliseconds to wait"=6) -> (w1228:cluster{i32, "milliseconds to wait":i32})  [unwired: 1 in]
    n1099 = property on="Buv Table" class="MCListbox (strict)"("ActiveCell"=w1232, "CellBG"=u32 16777226) -> ()  [unwired: 2 in, 2 out]
    n1100 = property on="Buv Table" class="MCListbox (strict)"("ActiveCell"=w1229, "CellBG"=u32 16777226) -> ()  [unwired: 2 in, 2 out]
    n1101 = property on="Buv Table" class="MCListbox (strict)"("ActiveCell"=w1228, "CellBG"=u32 16777226) -> ()  [unwired: 2 in, 2 out]
    n1102 = Bundle(w1215, 0) -> (w1222:cluster{i32, i32})  [unwired: 1 in]
    n1103 = property on="Buv Table" class="MCListbox (strict)"("ActiveCell"=w1222, "CellFont"=T7 {"Font Name"="Application font", "Size"=27, "Bold"=FALSE, "Italic"=FALSE, "Underline"=FALSE, "Strikeout"=FALSE, "Color"=0} ("Active Cell:Cell Font")) -> (error out=w1220:errorcluster)  [unwired: 2 in, 1 out]
    n1104 = Bundle(w1215, 1) -> (w1218:cluster{i32, i32})  [unwired: 1 in]
    n1105 = property on="Buv Table" class="MCListbox (strict)"(error in=w1220, "ActiveCell"=w1218, "CellFont"=w1214) -> ()  [unwired: 1 in, 2 out]
    n1106 = Bundle(w1215, 3) -> (w1217:cluster{i32, i32})  [unwired: 1 in]
    n1107 = property on="Buv Table" class="MCListbox (strict)"("ActiveCell"=w1217, "CellFont"=w1214) -> ()  [unwired: 2 in, 2 out]
  }
  n1108 = for "инициализация цветов и размера ячеек табл." {
    N: 50 -> [_]
    i -> [w1235]
    # "Линзы пост. тока"
    n1109 = flat-sequence {
      tunnel: w1235 -> [w1240]
      tunnel: [w1240] -> w1234
      tunnel: w1234 -> [w1279]
      tunnel: [w1279] -> w1233
      tunnel: w1233 -> [w1292]
      frame #0 {
        w1236 = "Application font" ("Font Name")
        n1110 = Bundle(w1240, 4) -> (w1252:cluster{i32, i32})  [unwired: 1 in]
        n1111 = property on="active" class="MCListbox (strict)"("ActiveCell"=w1252, "Height"=u32 35 ("Active Cell:Cell Size:Height"), "CellFontSize"=u16 28 ("Size")) -> ()  [unwired: 2 in, 2 out]
        n1112 = Bundle(w1240, 0) -> (w1263:cluster{i32, i32})  [unwired: 1 in]
        n1113 = Bundle(w1240, 2) -> (w1239:cluster{i32, i32})  [unwired: 1 in]
        n1114 = Bundle(w1240, 3) -> (w1253:cluster{i32, i32})  [unwired: 1 in]
        n1115 = Bundle(w1240, 1) -> (w1262:cluster{i32, i32})  [unwired: 1 in]
        n1116 = Bundle(w1240, 6) -> (w1238:cluster{i32, i32})  [unwired: 1 in]
        n1117 = Bundle(w1240, 5) -> (w1237:cluster{i32, i32})  [unwired: 1 in]
        n1118 = property on="active" class="MCListbox (strict)"("ActiveCell"=w1263, "Height"=u32 35 ("Active Cell:Cell Size:Height"), "CellFontSize"=u16 28 ("Size"), "CellFontName"=w1236) -> ()  [unwired: 2 in, 2 out]
        n1119 = property on="active" class="MCListbox (strict)"("ActiveCell"=w1239, "Height"=u32 35 ("Active Cell:Cell Size:Height"), "CellFontSize"=u16 28 ("Size"), "CellFontName"=w1236) -> ()  [unwired: 2 in, 2 out]
        n1120 = property on="active" class="MCListbox (strict)"("ActiveCell"=w1253, "Height"=u32 35 ("Active Cell:Cell Size:Height"), "CellFontSize"=u16 28 ("Size"), "CellFontName"=w1236) -> ()  [unwired: 2 in, 2 out]
        n1121 = property on="active" class="MCListbox (strict)"("ActiveCell"=w1262, "Height"=u32 35 ("Active Cell:Cell Size:Height"), "CellFontSize"=u16 28 ("Size"), "CellFontName"=w1236) -> ()  [unwired: 2 in, 2 out]
        n1122 = property on="active" class="MCListbox (strict)"("ActiveCell"=w1238, "Height"=u32 35 ("Active Cell:Cell Size:Height"), "CellFontSize"=u16 28 ("Size"), "CellFontName"=w1236) -> ()  [unwired: 2 in, 2 out]
        n1123 = property on="active" class="MCListbox (strict)"("ActiveCell"=w1237, "Height"=u32 35 ("Active Cell:Cell Size:Height"), "CellFontSize"=u16 28 ("Size"), "CellFontName"=w1236) -> ()  [unwired: 2 in, 2 out]
      }
      frame #1 {
        w1275 = T7 {"Font Name"="Application font", "Size"=28, "Bold"=FALSE, "Italic"=FALSE, "Underline"=FALSE, "Strikeout"=FALSE, "Color"=6908265} ("Active Cell:Cell Font")
        w1270 = T7 {"Font Name"="Application font", "Size"=30, "Bold"=TRUE, "Italic"=FALSE, "Underline"=FALSE, "Strikeout"=FALSE, "Color"=2263842} ("Active Cell:Cell Font")
        n1124 = Bundle(w1279, 3) -> (w1266:cluster{i32, i32})  [unwired: 1 in]
        n1125 = Bundle(w1279, 2) -> (w1269:cluster{i32, i32})  [unwired: 1 in]
        n1126 = Bundle(w1279, 0) -> (w1277:cluster{i32, i32})  [unwired: 1 in]
        n1127 = Bundle(w1279, 5) -> (w1273:cluster{i32, i32})  [unwired: 1 in]
        n1128 = Bundle(w1279, 4) -> (w1272:cluster{i32, i32})  [unwired: 1 in]
        n1129 = property on="active" class="MCListbox (strict)"("ActiveCell"=w1266, "CellFont"=w1270) -> ()  [unwired: 2 in, 2 out]
        n1130 = property on="active" class="MCListbox (strict)"("ActiveCell"=w1269, "CellFont"=w1270) -> ()  [unwired: 2 in, 2 out]
        n1131 = property on="active" class="MCListbox (strict)"("ActiveCell"=w1277, "CellFont"=T7 {"Font Name"="Application font", "Size"=28, "Bold"=FALSE, "Italic"=FALSE, "Underline"=FALSE, "Strikeout"=FALSE, "Color"=0} ("Active Cell:Cell Font")) -> ()  [unwired: 2 in, 2 out]
        n1132 = property on="active" class="MCListbox (strict)"("ActiveCell"=w1273, "CellFont"=w1275) -> ()  [unwired: 2 in, 2 out]
        n1133 = property on="active" class="MCListbox (strict)"("ActiveCell"=w1272, "CellFont"=w1275) -> ()  [unwired: 2 in, 2 out]
      }
      frame #2 {
        w1291 = T7 {"Font Name"="Application font", "Size"=28, "Bold"=FALSE, "Italic"=FALSE, "Underline"=FALSE, "Strikeout"=FALSE, "Color"=0} ("Active Cell:Cell Font")
        n1134 = Bundle(w1292, 6) -> (w1286:cluster{i32, i32})  [unwired: 1 in]
        n1135 = Bundle(w1292, 8) -> (w1287:cluster{i32, i32})  [unwired: 1 in]
        n1136 = Bundle(w1292, 7) -> (w1288:cluster{i32, i32})  [unwired: 1 in]
        n1137 = property on="active" class="MCListbox (strict)"("ActiveCell"=w1286, "CellBG"=u32 16777225) -> (error out=w1285:errorcluster)  [unwired: 2 in, 1 out]
        n1138 = property on="error" class="MCListbox (strict)"("ActiveCell"=w1287, "CellBG"=u32 16777225) -> ()  [unwired: 2 in, 2 out]
        n1139 = property on="out" class="MCListbox (strict)"("ActiveCell"=w1288, "CellBG"=u32 16777225) -> (error out=w1289:errorcluster)  [unwired: 2 in, 1 out]
        n1140 = property on="active" class="MCListbox (strict)"(error in=w1285, "ActiveCell"=w1286, "CellFont"=w1291) -> ()  [unwired: 1 in, 2 out]
        n1141 = property on="active" class="MCListbox (strict)"(error in=w1289, "ActiveCell"=w1288, "CellFont"=w1291) -> ()  [unwired: 1 in, 2 out]
      }
    }
  }
  n1142 = Build Array(w4, w4, w4, w4, w4, w4, w4, w4) -> (w5:string[][])
  n1143 = local write "BuvCtrlVI_VIRef"(refnum<vi>[] [] ("BuvCtrlVI_VIRef")) -> ()
  n1144 = Transpose 2D Array(2D array=w5) -> (transposed array=w6:string[][])
  n1145 = property on="List of channels" class="MCListbox (strict)"("ItemNames"=w6) -> ()  [unwired: 2 in, 2 out]
  "Measure_VI" <- refnum<vi>[] []
  "ADRESS" <- string[] [] ("GlobalInAdress")
  "NAME" <- string[] [] ("GlobalInAdress")
  "CURRENTSET" <- dbl[] [] ("GlobalInAdress")
  "T upd fl" <- FALSE ("T upd fl")
